vi "RUN.vi"(8 "error in (no error)":errorcluster, 11 "SPARC4_AC in":refnum<class "S4ACS_GUI.lvclass">) -> (0 "error out":errorcluster, 3 "SPARC4_AC out":refnum<class "S4ACS_GUI.lvclass">)   [LabVIEW 2018, in "S4ACS_GUI.lvclass"]
uses:
  S4ACS_GUI.lvclass
  StateMachine/State Machine.lvclass
  Interface/Interface.lvclass
  RxTx/RxTx.lvclass
  SyncBox/Sync Box.lvclass
  Channel Manager/Channel Manager.lvclass
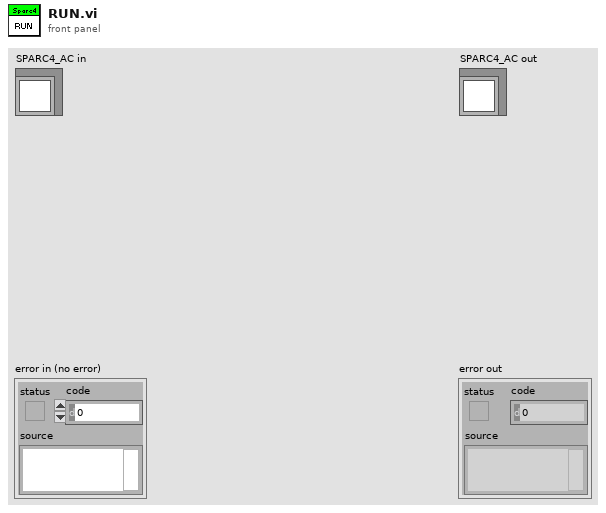
[diagram p1: front panel]
types:
  T1 = cluster{"Image Name":string, "Image Path":string, "# Images":u32, "Exposure Time":dbl, "Pre-amp gain":u8, "Readout Rate":u8, "Vertical Shift Speed":u8, "Acquisition Mode":u8, "Trigger":u8, "Read Mode":u8, "EM Mode":u8, "EM Gain":u16, "Shutter Mode":u8, "Shutter TTL":u8, "Time to open shutter":u16, "Time to close shutter":u16, "Vertical Binning":u16, "Horizontal Binning":u16, "Initial Line":u16, "Initial Column":u16, "Final Line":u16, "Final Column":u16, "Image Name (TEMP)":string, "#img in sequence":u32, "Kinetic Series Length":u32, "Number of Accumulations":u32, "Kinetic Cycle Time":u32, "Frame Transfer":bool, "Vertical Clock Amplitude":u8}
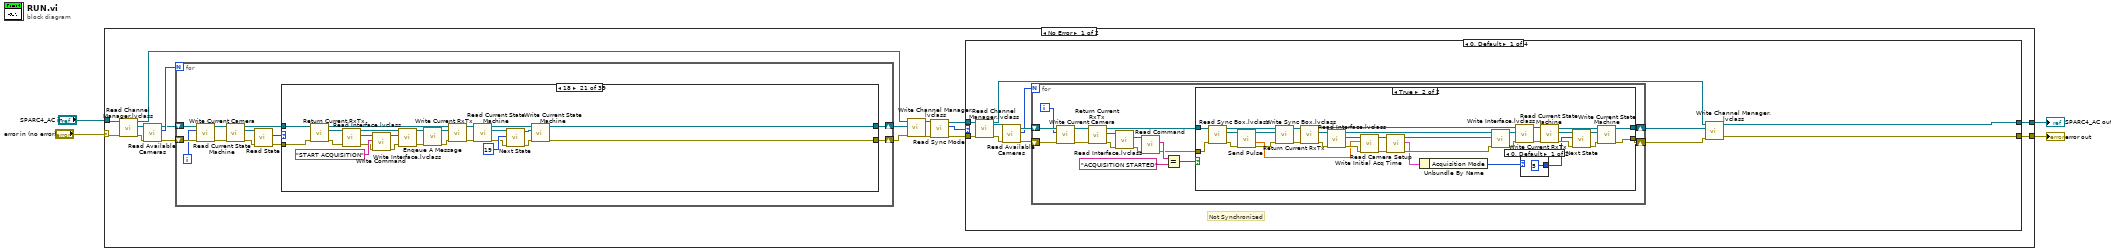
[diagram p0: block diagram]
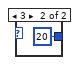
[diagram p3: hidden frame]
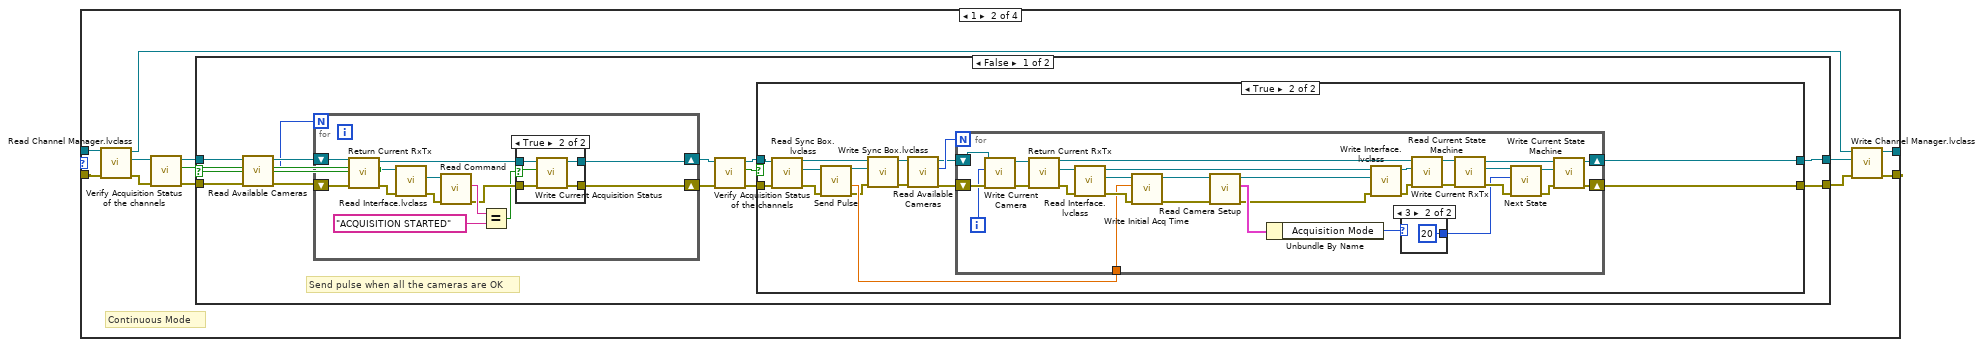
[diagram p4: hidden frame]
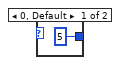
[diagram p6: hidden frame]
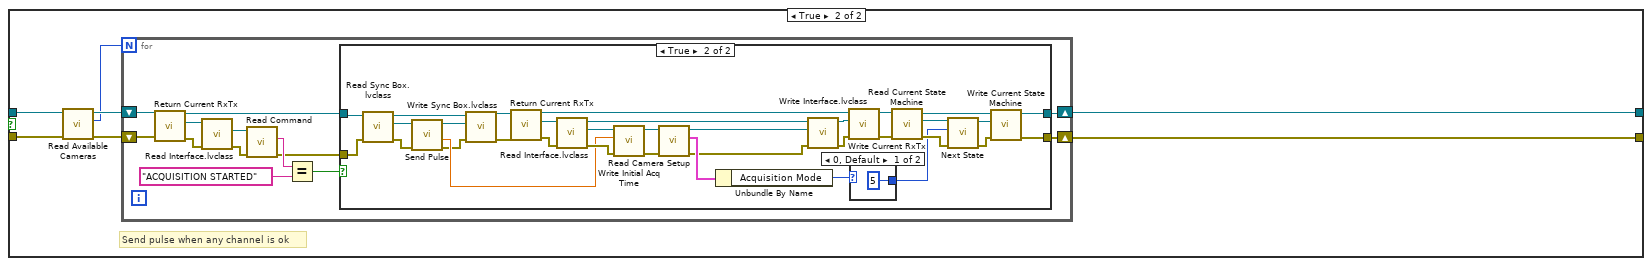
[diagram p8: hidden frame]
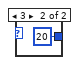
[diagram p10: hidden frame]
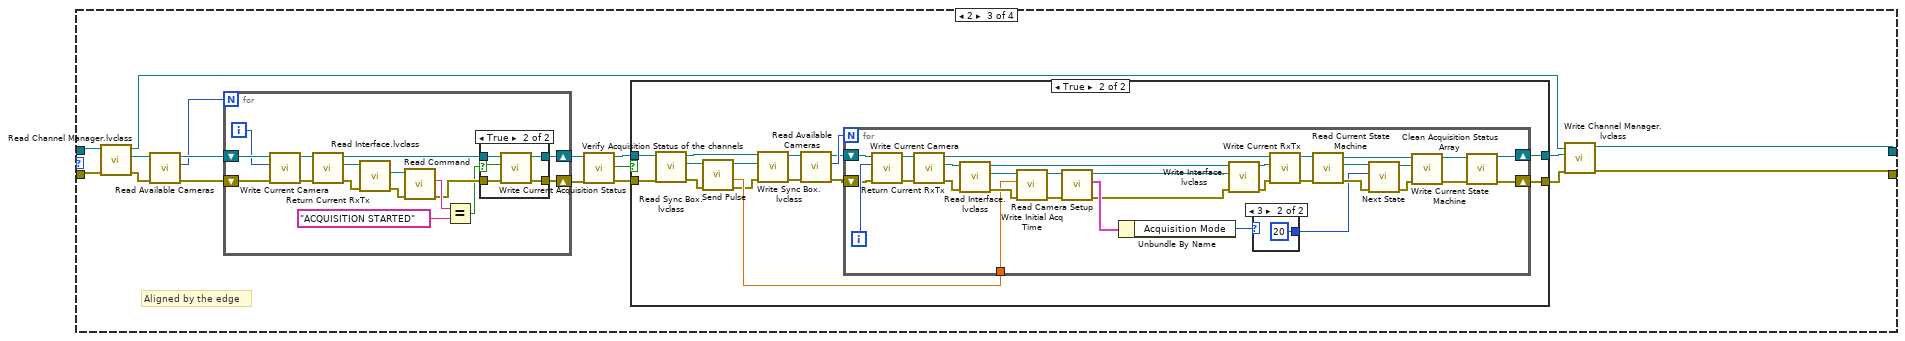
[diagram p11: hidden frame]
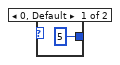
[diagram p13: hidden frame]
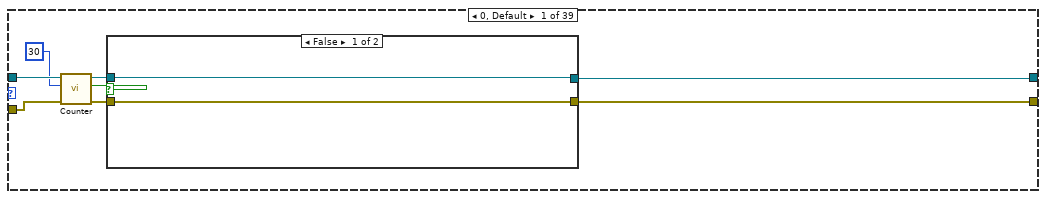
[diagram p16: hidden frame]
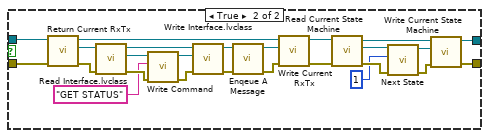
[diagram p17: hidden frame]
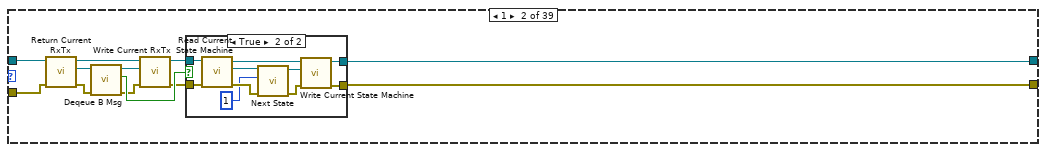
[diagram p18: hidden frame]
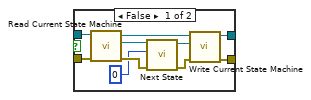
[diagram p19: hidden frame]
diagram:
  n1 = case shown="No Error" "error in (no error)" {
    selector: "error in (no error)" -> [w21 w1413]
    tunnel: [w16 w1414] -> w2
    tunnel: "SPARC4_AC in" -> [w20 w1414]
    tunnel: [w15 w1413] -> w1
    frame No Error {
      n2 = call-dynamic "Read Channel Manager.lvclass.vi"("error in (no error)"=w21, "SPARC4_AC in"=w20) -> ("error out"=w8:errorcluster, "Channel Manager.lvclass"=w9:refnum<class "Channel Manager.lvclass">, "SPARC4_AC out"=w12:refnum<class "S4ACS_GUI.lvclass">)  [unwired: 7 in]
      n3 = call-dynamic "Read Available Cameras.vi"("error in (no error)"=w8, "Channel Manager in"=w9) -> ("error out"=w5:errorcluster, "Available Cameras"=w7:u8, "Channel Manager out"=w6:refnum<class "Channel Manager.lvclass">)  [unwired: 7 in]
      n4 = for {
        N: w7 -> [_]
        shift-right: [w337] -> w13
        shift-left: w6 -> [w334]
        shift-right: [w338] -> w14
        shift-left: w5 -> [w333]
        i -> [w332]
        n5 = call-dynamic "Write Current Camera.vi"("error in (no error)"=w333, "Current Camera"=w332, "Channel Manager in"=w334) -> ("error out"=w336:errorcluster, "Channel Manager out"=w335:refnum<class "Channel Manager.lvclass">)  [unwired: 7 in]
        n6 = call "Read Current State Machine.vi"("error in (no error)"=w336, "Channel Manager in"=w335) -> ("error out"=w340:errorcluster, "State Machine.lvclass"=w341:refnum<class "State Machine.lvclass">, "Channel Manager out"=w339:refnum<class "Channel Manager.lvclass">)  [unwired: 7 in]
        n7 = call-dynamic "Read State.vi"("error in (no error)"=w340, "State Machine in"=w341) -> ("error out"=w342:errorcluster, "State"=w343:u8)  [unwired: 7 in, 1 out]
        n8 = case shown="18" w343 {
          tunnel: w342 -> [w349 w389 w411 w429 w451 w468 w506 w520 w573 w598 w655 w665 w706 w724 w746 w771 w815 w830 w858 w863 w890 w915 w948 w974 w998 w1024 w1049 w1073 w1108 w1145 w1188 w1198 w1227 w1263 w1286 w1305 w1342 w1366 w1391]
          tunnel: w339 -> [w346 w390 w412 w430 w450 w467 w507 w521 w574 w597 w656 w664 w707 w725 w747 w772 w816 w831 w859 w862 w889 w914 w947 w973 w999 w1023 w1050 w1072 w1109 w1146 w1187 w1197 w1228 w1262 w1287 w1306 w1343 w1367 w1392]
          tunnel: [w351 w380 w412 w414 w440 w465 w493 w516 w560 w596 w644 w662 w698 w714 w733 w770 w804 w828 w859 w861 w888 w913 w937 w972 w997 w1022 w1047 w1071 w1107 w1144 w1186 w1196 w1226 w1261 w1285 w1304 w1341 w1365 w1390] -> w337
          tunnel: [w350 w379 w411 w413 w441 w466 w492 w515 w559 w595 w643 w663 w697 w713 w732 w769 w803 w827 w858 w860 w887 w912 w923 w971 w996 w1021 w1048 w1070 w1106 w1143 w1185 w1195 w1225 w1260 w1284 w1303 w1340 w1364 w1389] -> w338
          frame 0, Default {
            n9 = call "Counter.vi"("error in (no error)"=w349, "Interval"=u16 30, "Channel Manager in"=w346) -> ("error out"=w348:errorcluster, "Timeout?"=w345:bool, "Channel Manager out"=w347:refnum<class "Channel Manager.lvclass">)  [unwired: 6 in]
            n10 = case shown="False" w345 {
              tunnel: [w353 w357] -> w351
              tunnel: [w352 w356] -> w350
              tunnel: w348 -> [w352 w355]
              tunnel: w347 -> [w353 w354]
              frame False {
              }
              frame True {
                n11 = call "Return Current RxTx.vi"("error in (no error)"=w355, "Channel Manager in"=w354) -> ("error out"=w369:errorcluster, "RxTx"=w370:refnum<class "RxTx.lvclass">, "Channel Manager out"=w368:refnum<class "Channel Manager.lvclass">)  [unwired: 7 in]
                n12 = call-dynamic "Read Interface.lvclass.vi"("error in (no error)"=w369, "RxTx in"=w370) -> ("error out"=w377:errorcluster, "Interface.lvclass"=w378:refnum<class "Interface.lvclass">, "RxTx out"=w374:refnum<class "RxTx.lvclass">)  [unwired: 7 in]
                n13 = call "Write Command.vi"("error in (no error)"=w377, "Command"="GET STATUS", "Interface in"=w378) -> ("error out"=w376:errorcluster, "Interface out"=w375:refnum<class "Interface.lvclass">)  [unwired: 7 in]
                n14 = call-dynamic "Write Interface.lvclass.vi"("error in (no error)"=w376, "Interface.lvclass"=w375, "RxTx in"=w374) -> ("error out"=w372:errorcluster, "RxTx out"=w371:refnum<class "RxTx.lvclass">)  [unwired: 7 in]
                n15 = call "Enqeue A Message.vi"("error in (no error)"=w372, "RxTx in"=w371) -> ("error out"=w366:errorcluster, "RxTx out"=w367:refnum<class "RxTx.lvclass">)  [unwired: 8 in]
                n16 = call "Write Current RxTx.vi"("error in (no error)"=w366, "RxTx"=w367, "Channel Manager in"=w368) -> ("error out"=w359:errorcluster, "Channel Manager out"=w358:refnum<class "Channel Manager.lvclass">)  [unwired: 7 in]
                n17 = call "Read Current State Machine.vi"("error in (no error)"=w359, "Channel Manager in"=w358) -> ("error out"=w361:errorcluster, "State Machine.lvclass"=w362:refnum<class "State Machine.lvclass">, "Channel Manager out"=w365:refnum<class "Channel Manager.lvclass">)  [unwired: 7 in]
                n18 = call "Next State.vi"("error in (no error)"=w361, "New_State"=u32 1, "State Machine in"=w362) -> ("error out"=w363:errorcluster, "State Machine out"=w364:refnum<class "State Machine.lvclass">)  [unwired: 7 in]
                n19 = call "Write Current State Machine.vi"("error in (no error)"=w363, "State Machine.lvclass"=w364, "Channel Manager in"=w365) -> ("error out"=w356:errorcluster, "Channel Manager out"=w357:refnum<class "Channel Manager.lvclass">)  [unwired: 7 in]
              }
            }
          }
          frame 1 {
            n20 = call "Return Current RxTx.vi"("error in (no error)"=w389, "Channel Manager in"=w390) -> ("error out"=w387:errorcluster, "RxTx"=w388:refnum<class "RxTx.lvclass">, "Channel Manager out"=w383:refnum<class "Channel Manager.lvclass">)  [unwired: 7 in]
            n21 = call "Deqeue B Msg.vi"("error in (no error)"=w387, "RxTx in"=w388) -> ("error out"=w385:errorcluster, "timeout?"=w386:bool, "RxTx out"=w384:refnum<class "RxTx.lvclass">)  [unwired: 7 in]
            n22 = call "Write Current RxTx.vi"("error in (no error)"=w385, "RxTx"=w384, "Channel Manager in"=w383) -> ("error out"=w381:errorcluster, "Channel Manager out"=w382:refnum<class "Channel Manager.lvclass">)  [unwired: 7 in]
            n23 = case shown="True" w386 {
              tunnel: w382 -> [w393 w404]
              tunnel: w381 -> [w394 w403]
              tunnel: [w392 w402] -> w380
              tunnel: [w391 w401] -> w379
              frame False {
                n24 = call "Read Current State Machine.vi"("error in (no error)"=w394, "Channel Manager in"=w393) -> ("error out"=w396:errorcluster, "State Machine.lvclass"=w397:refnum<class "State Machine.lvclass">, "Channel Manager out"=w400:refnum<class "Channel Manager.lvclass">)  [unwired: 7 in]
                n25 = call "Next State.vi"("error in (no error)"=w396, "New_State"=u32 0, "State Machine in"=w397) -> ("error out"=w398:errorcluster, "State Machine out"=w399:refnum<class "State Machine.lvclass">)  [unwired: 7 in]
                n26 = call "Write Current State Machine.vi"("error in (no error)"=w398, "State Machine.lvclass"=w399, "Channel Manager in"=w400) -> ("error out"=w391:errorcluster, "Channel Manager out"=w392:refnum<class "Channel Manager.lvclass">)  [unwired: 7 in]
              }
              frame True {
                n27 = call "Read Current State Machine.vi"("error in (no error)"=w403, "Channel Manager in"=w404) -> ("error out"=w406:errorcluster, "State Machine.lvclass"=w407:refnum<class "State Machine.lvclass">, "Channel Manager out"=w410:refnum<class "Channel Manager.lvclass">)  [unwired: 7 in]
                n28 = call "Next State.vi"("error in (no error)"=w406, "New_State"=u32 1, "State Machine in"=w407) -> ("error out"=w408:errorcluster, "State Machine out"=w409:refnum<class "State Machine.lvclass">)  [unwired: 7 in]
                n29 = call "Write Current State Machine.vi"("error in (no error)"=w408, "State Machine.lvclass"=w409, "Channel Manager in"=w410) -> ("error out"=w401:errorcluster, "Channel Manager out"=w402:refnum<class "Channel Manager.lvclass">)  [unwired: 7 in]
              }
            }
          }
          frame 99 {
          }
          frame 2 {
            # "Limpa array de status de aquisição.\nNecessário para o modo de sincronização contínuo"
            n30 = call "Return Current RxTx.vi"("error in (no error)"=w429, "Channel Manager in"=w430) -> ("error out"=w427:errorcluster, "RxTx"=w428:refnum<class "RxTx.lvclass">, "Channel Manager out"=w424:refnum<class "Channel Manager.lvclass">)  [unwired: 7 in]
            n31 = call-dynamic "Read Interface.lvclass.vi"("error in (no error)"=w427, "RxTx in"=w428) -> ("error out"=w437:errorcluster, "Interface.lvclass"=w438:refnum<class "Interface.lvclass">, "RxTx out"=w432:refnum<class "RxTx.lvclass">)  [unwired: 7 in]
            n32 = call "Write Command.vi"("error in (no error)"=w437, "Command"="WRITE CAMERA SETUP", "Interface in"=w438) -> ("error out"=w434:errorcluster, "Interface out"=w433:refnum<class "Interface.lvclass">)  [unwired: 7 in]
            n33 = call-dynamic "Write Interface.lvclass.vi"("error in (no error)"=w434, "Interface.lvclass"=w433, "RxTx in"=w432) -> ("error out"=w436:errorcluster, "RxTx out"=w435:refnum<class "RxTx.lvclass">)  [unwired: 7 in]
            n34 = call "Enqeue A Message.vi"("error in (no error)"=w436, "RxTx in"=w435) -> ("error out"=w426:errorcluster, "RxTx out"=w425:refnum<class "RxTx.lvclass">)  [unwired: 8 in]
            n35 = call "Write Current RxTx.vi"("error in (no error)"=w426, "RxTx"=w425, "Channel Manager in"=w424) -> ("error out"=w423:errorcluster, "Channel Manager out"=w422:refnum<class "Channel Manager.lvclass">)  [unwired: 7 in]
            n36 = call "Read Current State Machine.vi"("error in (no error)"=w423, "Channel Manager in"=w422) -> ("error out"=w420:errorcluster, "State Machine.lvclass"=w421:refnum<class "State Machine.lvclass">, "Channel Manager out"=w417:refnum<class "Channel Manager.lvclass">)  [unwired: 7 in]
            n37 = call "Next State.vi"("error in (no error)"=w420, "New_State"=u32 3, "State Machine in"=w421) -> ("error out"=w419:errorcluster, "State Machine out"=w418:refnum<class "State Machine.lvclass">)  [unwired: 7 in]
            n38 = call "Write Current State Machine.vi"("error in (no error)"=w419, "State Machine.lvclass"=w418, "Channel Manager in"=w417) -> ("error out"=w416:errorcluster, "Channel Manager out"=w415:refnum<class "Channel Manager.lvclass">)  [unwired: 7 in]
            n39 = call "Clean Acquisition Status Array.vi"("error in (no error)"=w416, "Channel Manager in"=w415) -> ("error out"=w413:errorcluster, "Channel Manager out"=w414:refnum<class "Channel Manager.lvclass">)  [unwired: 8 in]
          }
          frame 3 {
            n40 = call "Return Current RxTx.vi"("error in (no error)"=w451, "Channel Manager in"=w450) -> ("error out"=w455:errorcluster, "RxTx"=w456:refnum<class "RxTx.lvclass">, "Channel Manager out"=w452:refnum<class "Channel Manager.lvclass">)  [unwired: 7 in]
            n41 = call-dynamic "Read Interface.lvclass.vi"("error in (no error)"=w455, "RxTx in"=w456) -> ("error out"=w462:errorcluster, "Interface.lvclass"=w463:refnum<class "Interface.lvclass">, "RxTx out"=w457:refnum<class "RxTx.lvclass">)  [unwired: 7 in]
            n42 = call "Write Command.vi"("error in (no error)"=w462, "Command"="START ACQUISITION", "Interface in"=w463) -> ("error out"=w459:errorcluster, "Interface out"=w458:refnum<class "Interface.lvclass">)  [unwired: 7 in]
            n43 = call-dynamic "Write Interface.lvclass.vi"("error in (no error)"=w459, "Interface.lvclass"=w458, "RxTx in"=w457) -> ("error out"=w461:errorcluster, "RxTx out"=w460:refnum<class "RxTx.lvclass">)  [unwired: 7 in]
            n44 = call "Enqeue A Message.vi"("error in (no error)"=w461, "RxTx in"=w460) -> ("error out"=w454:errorcluster, "RxTx out"=w453:refnum<class "RxTx.lvclass">)  [unwired: 8 in]
            n45 = call "Write Current RxTx.vi"("error in (no error)"=w454, "RxTx"=w453, "Channel Manager in"=w452) -> ("error out"=w444:errorcluster, "Channel Manager out"=w443:refnum<class "Channel Manager.lvclass">)  [unwired: 7 in]
            n46 = call "Read Current State Machine.vi"("error in (no error)"=w444, "Channel Manager in"=w443) -> ("error out"=w448:errorcluster, "State Machine.lvclass"=w447:refnum<class "State Machine.lvclass">, "Channel Manager out"=w442:refnum<class "Channel Manager.lvclass">)  [unwired: 7 in]
            n47 = call "Next State.vi"("error in (no error)"=w448, "New_State"=u32 4, "State Machine in"=w447) -> ("error out"=w446:errorcluster, "State Machine out"=w445:refnum<class "State Machine.lvclass">)  [unwired: 7 in]
            n48 = call "Write Current State Machine.vi"("error in (no error)"=w446, "State Machine.lvclass"=w445, "Channel Manager in"=w442) -> ("error out"=w441:errorcluster, "Channel Manager out"=w440:refnum<class "Channel Manager.lvclass">)  [unwired: 7 in]
          }
          frame 4 {
            n49 = call "Return Current RxTx.vi"("error in (no error)"=w468, "Channel Manager in"=w467) -> ("error out"=w472:errorcluster, "RxTx"=w473:refnum<class "RxTx.lvclass">, "Channel Manager out"=w474:refnum<class "Channel Manager.lvclass">)  [unwired: 7 in]
            n50 = call "Deqeue B Msg.vi"("error in (no error)"=w472, "RxTx in"=w473) -> ("error out"=w475:errorcluster, "timeout?"=w469:bool, "RxTx out"=w476:refnum<class "RxTx.lvclass">)  [unwired: 7 in]
            n51 = call "Write Current RxTx.vi"("error in (no error)"=w475, "RxTx"=w476, "Channel Manager in"=w474) -> ("error out"=w471:errorcluster, "Channel Manager out"=w470:refnum<class "Channel Manager.lvclass">)  [unwired: 7 in]
            n52 = case shown="True" w469 {
              tunnel: w471 -> [w477 w482]
              tunnel: w470 -> [w478 w481]
              tunnel: [w478 w480] -> w465
              tunnel: [w477 w479] -> w466
              frame False {
              }
              frame True {
                n53 = call "Read Current State Machine.vi"("error in (no error)"=w482, "Channel Manager in"=w481) -> ("error out"=w484:errorcluster, "State Machine.lvclass"=w485:refnum<class "State Machine.lvclass">, "Channel Manager out"=w488:refnum<class "Channel Manager.lvclass">)  [unwired: 7 in]
                n54 = call "Next State.vi"("error in (no error)"=w484, "New_State"=u32 4, "State Machine in"=w485) -> ("error out"=w486:errorcluster, "State Machine out"=w487:refnum<class "State Machine.lvclass">)  [unwired: 7 in]
                n55 = call "Write Current State Machine.vi"("error in (no error)"=w486, "State Machine.lvclass"=w487, "Channel Manager in"=w488) -> ("error out"=w479:errorcluster, "Channel Manager out"=w480:refnum<class "Channel Manager.lvclass">)  [unwired: 7 in]
              }
            }
          }
          frame 5 {
            n56 = call "Return Current RxTx.vi"("error in (no error)"=w506, "Channel Manager in"=w507) -> ("error out"=w504:errorcluster, "RxTx"=w505:refnum<class "RxTx.lvclass">, "Channel Manager out"=w501:refnum<class "Channel Manager.lvclass">)  [unwired: 7 in]
            n57 = call-dynamic "Read Interface.lvclass.vi"("error in (no error)"=w504, "RxTx in"=w505) -> ("error out"=w512:errorcluster, "Interface.lvclass"=w513:refnum<class "Interface.lvclass">, "RxTx out"=w509:refnum<class "RxTx.lvclass">)  [unwired: 7 in]
            n58 = call "Write Command.vi"("error in (no error)"=w512, "Command"="VERIFY ACQUISITION", "Interface in"=w513) -> ("error out"=w490:errorcluster, "Interface out"=w491:refnum<class "Interface.lvclass">)  [unwired: 7 in]
            n59 = call-dynamic "Write Interface.lvclass.vi"("error in (no error)"=w490, "Interface.lvclass"=w491, "RxTx in"=w509) -> ("error out"=w511:errorcluster, "RxTx out"=w510:refnum<class "RxTx.lvclass">)  [unwired: 7 in]
            n60 = call "Enqeue A Message.vi"("error in (no error)"=w511, "RxTx in"=w510) -> ("error out"=w503:errorcluster, "RxTx out"=w502:refnum<class "RxTx.lvclass">)  [unwired: 8 in]
            n61 = call "Write Current RxTx.vi"("error in (no error)"=w503, "RxTx"=w502, "Channel Manager in"=w501) -> ("error out"=w500:errorcluster, "Channel Manager out"=w499:refnum<class "Channel Manager.lvclass">)  [unwired: 7 in]
            n62 = call "Read Current State Machine.vi"("error in (no error)"=w500, "Channel Manager in"=w499) -> ("error out"=w498:errorcluster, "State Machine.lvclass"=w497:refnum<class "State Machine.lvclass">, "Channel Manager out"=w494:refnum<class "Channel Manager.lvclass">)  [unwired: 7 in]
            n63 = call "Next State.vi"("error in (no error)"=w498, "New_State"=u32 6, "State Machine in"=w497) -> ("error out"=w496:errorcluster, "State Machine out"=w495:refnum<class "State Machine.lvclass">)  [unwired: 7 in]
            n64 = call "Write Current State Machine.vi"("error in (no error)"=w496, "State Machine.lvclass"=w495, "Channel Manager in"=w494) -> ("error out"=w492:errorcluster, "Channel Manager out"=w493:refnum<class "Channel Manager.lvclass">)  [unwired: 7 in]
          }
          frame 6 {
            n65 = call "Return Current RxTx.vi"("error in (no error)"=w520, "Channel Manager in"=w521) -> ("error out"=w518:errorcluster, "RxTx"=w519:refnum<class "RxTx.lvclass">, "Channel Manager out"=w517:refnum<class "Channel Manager.lvclass">)  [unwired: 7 in]
            n66 = call "Deqeue B Msg.vi"("error in (no error)"=w518, "RxTx in"=w519) -> ("error out"=w523:errorcluster, "timeout?"=w514:bool, "RxTx out"=w522:refnum<class "RxTx.lvclass">)  [unwired: 7 in]
            n67 = case shown="False" w514 {
              tunnel: w523 -> [w541 w553]
              tunnel: w522 -> [w540 w552]
              tunnel: w517 -> [w535 w551]
              tunnel: [w527 w548] -> w516
              tunnel: [w526 w547] -> w515
              frame False {
                n68 = call-dynamic "Read Interface.lvclass.vi"("error in (no error)"=w541, "RxTx in"=w540) -> ("error out"=w538:errorcluster, "Interface.lvclass"=w539:refnum<class "Interface.lvclass">, "RxTx out"=w537:refnum<class "RxTx.lvclass">)  [unwired: 7 in]
                n69 = call "Read Command.vi"("error in (no error)"=w538, "Interface in"=w539) -> ("error out"=w536:errorcluster, "Command"=w525:string)  [unwired: 7 in, 1 out]
                n70 = call "Write Current RxTx.vi"("error in (no error)"=w536, "RxTx"=w537, "Channel Manager in"=w535) -> ("error out"=w534:errorcluster, "Channel Manager out"=w533:refnum<class "Channel Manager.lvclass">)  [unwired: 7 in]
                n71 = case shown="\"ACQUISITION COMPLETED\"" w525 {
                  tunnel: [u32 4 ("New_State") u32 7 ("New_State") u32 9 ("New_State")] -> w524
                  frame "False", Default {
                  }
                  frame "ACQUIRING" {
                  }
                  frame "ACQUISITION COMPLETED" {
                  }
                }
                n72 = call "Read Current State Machine.vi"("error in (no error)"=w534, "Channel Manager in"=w533) -> ("error out"=w531:errorcluster, "State Machine.lvclass"=w532:refnum<class "State Machine.lvclass">, "Channel Manager out"=w528:refnum<class "Channel Manager.lvclass">)  [unwired: 7 in]
                n73 = call "Next State.vi"("error in (no error)"=w531, "New_State"=w524, "State Machine in"=w532) -> ("error out"=w530:errorcluster, "State Machine out"=w529:refnum<class "State Machine.lvclass">)  [unwired: 7 in]
                n74 = call "Write Current State Machine.vi"("error in (no error)"=w530, "State Machine.lvclass"=w529, "Channel Manager in"=w528) -> ("error out"=w526:errorcluster, "Channel Manager out"=w527:refnum<class "Channel Manager.lvclass">)  [unwired: 7 in]
              }
              frame True {
                n75 = call "Write Current RxTx.vi"("error in (no error)"=w553, "RxTx"=w552, "Channel Manager in"=w551) -> ("error out"=w550:errorcluster, "Channel Manager out"=w549:refnum<class "Channel Manager.lvclass">)  [unwired: 7 in]
                n76 = call "Read Current State Machine.vi"("error in (no error)"=w550, "Channel Manager in"=w549) -> ("error out"=w546:errorcluster, "State Machine.lvclass"=w556:refnum<class "State Machine.lvclass">, "Channel Manager out"=w554:refnum<class "Channel Manager.lvclass">)  [unwired: 7 in]
                n77 = call "Next State.vi"("error in (no error)"=w546, "New_State"=u32 6, "State Machine in"=w556) -> ("error out"=w557:errorcluster, "State Machine out"=w555:refnum<class "State Machine.lvclass">)  [unwired: 7 in]
                n78 = call "Write Current State Machine.vi"("error in (no error)"=w557, "State Machine.lvclass"=w555, "Channel Manager in"=w554) -> ("error out"=w547:errorcluster, "Channel Manager out"=w548:refnum<class "Channel Manager.lvclass">)  [unwired: 7 in]
              }
            }
          }
          frame 7 {
            n79 = call "Return Current RxTx.vi"("error in (no error)"=w573, "Channel Manager in"=w574) -> ("error out"=w571:errorcluster, "RxTx"=w572:refnum<class "RxTx.lvclass">, "Channel Manager out"=w562:refnum<class "Channel Manager.lvclass">)  [unwired: 7 in]
            n80 = call-dynamic "Read Interface.lvclass.vi"("error in (no error)"=w571, "RxTx in"=w572) -> ("error out"=w579:errorcluster, "Interface.lvclass"=w580:refnum<class "Interface.lvclass">, "RxTx out"=w575:refnum<class "RxTx.lvclass">)  [unwired: 7 in]
            n81 = call-dynamic "Read Abort.vi"("error in (no error)"=w579, "Interface in"=w580) -> ("error out"=w576:errorcluster, "Abort"=w578:bool, "Interface out"=w577:refnum<class "Interface.lvclass">)  [unwired: 7 in]
            n82 = case shown="False" w578 {
              tunnel: w577 -> [_ w593]
              tunnel: w576 -> [w582 w592]
              tunnel: w575 -> [w583 w589]
              tunnel: [w583 w586] -> w563
              tunnel: [w582 w585] -> w561
              tunnel: [5 8] -> w558
              frame False {
              }
              frame True {
                n83 = call "Write Command.vi"("error in (no error)"=w592, "Command"="ABORT ACQUISITION", "Interface in"=w593) -> ("error out"=w588:errorcluster, "Interface out"=w587:refnum<class "Interface.lvclass">)  [unwired: 7 in]
                n84 = call-dynamic "Write Interface.lvclass.vi"("error in (no error)"=w588, "Interface.lvclass"=w587, "RxTx in"=w589) -> ("error out"=w590:errorcluster, "RxTx out"=w591:refnum<class "RxTx.lvclass">)  [unwired: 7 in]
                n85 = call "Enqeue A Message.vi"("error in (no error)"=w590, "RxTx in"=w591) -> ("error out"=w585:errorcluster, "RxTx out"=w586:refnum<class "RxTx.lvclass">)  [unwired: 8 in]
              }
            }
            n86 = call "Write Current RxTx.vi"("error in (no error)"=w561, "RxTx"=w563, "Channel Manager in"=w562) -> ("error out"=w570:errorcluster, "Channel Manager out"=w569:refnum<class "Channel Manager.lvclass">)  [unwired: 7 in]
            n87 = call "Read Current State Machine.vi"("error in (no error)"=w570, "Channel Manager in"=w569) -> ("error out"=w567:errorcluster, "State Machine.lvclass"=w568:refnum<class "State Machine.lvclass">, "Channel Manager out"=w564:refnum<class "Channel Manager.lvclass">)  [unwired: 7 in]
            n88 = call "Next State.vi"("error in (no error)"=w567, "New_State"=w558, "State Machine in"=w568) -> ("error out"=w566:errorcluster, "State Machine out"=w565:refnum<class "State Machine.lvclass">)  [unwired: 7 in]
            n89 = call "Write Current State Machine.vi"("error in (no error)"=w566, "State Machine.lvclass"=w565, "Channel Manager in"=w564) -> ("error out"=w559:errorcluster, "Channel Manager out"=w560:refnum<class "Channel Manager.lvclass">)  [unwired: 7 in]
          }
          frame 8 {
            n90 = call "Return Current RxTx.vi"("error in (no error)"=w598, "Channel Manager in"=w597) -> ("error out"=w605:errorcluster, "RxTx"=w606:refnum<class "RxTx.lvclass">, "Channel Manager out"=w601:refnum<class "Channel Manager.lvclass">)  [unwired: 7 in]
            n91 = call "Deqeue B Msg.vi"("error in (no error)"=w605, "RxTx in"=w606) -> ("error out"=w603:errorcluster, "timeout?"=w604:bool, "RxTx out"=w602:refnum<class "RxTx.lvclass">)  [unwired: 7 in]
            n92 = call "Write Current RxTx.vi"("error in (no error)"=w603, "RxTx"=w602, "Channel Manager in"=w601) -> ("error out"=w599:errorcluster, "Channel Manager out"=w600:refnum<class "Channel Manager.lvclass">)  [unwired: 7 in]
            n93 = case shown="False" w604 {
              tunnel: w600 -> [w609 w620]
              tunnel: w599 -> [w610 w619]
              tunnel: [w608 w618] -> w596
              tunnel: [w607 w617] -> w595
              frame False {
                n94 = call "Read Current State Machine.vi"("error in (no error)"=w610, "Channel Manager in"=w609) -> ("error out"=w612:errorcluster, "State Machine.lvclass"=w613:refnum<class "State Machine.lvclass">, "Channel Manager out"=w616:refnum<class "Channel Manager.lvclass">)  [unwired: 7 in]
                n95 = call "Next State.vi"("error in (no error)"=w612, "New_State"=u32 0, "State Machine in"=w613) -> ("error out"=w614:errorcluster, "State Machine out"=w615:refnum<class "State Machine.lvclass">)  [unwired: 7 in]
                n96 = call "Write Current State Machine.vi"("error in (no error)"=w614, "State Machine.lvclass"=w615, "Channel Manager in"=w616) -> ("error out"=w607:errorcluster, "Channel Manager out"=w608:refnum<class "Channel Manager.lvclass">)  [unwired: 7 in]
              }
              frame True {
                n97 = call "Read Current State Machine.vi"("error in (no error)"=w619, "Channel Manager in"=w620) -> ("error out"=w622:errorcluster, "State Machine.lvclass"=w623:refnum<class "State Machine.lvclass">, "Channel Manager out"=w626:refnum<class "Channel Manager.lvclass">)  [unwired: 7 in]
                n98 = call "Next State.vi"("error in (no error)"=w622, "New_State"=u32 8, "State Machine in"=w623) -> ("error out"=w624:errorcluster, "State Machine out"=w625:refnum<class "State Machine.lvclass">)  [unwired: 7 in]
                n99 = call "Write Current State Machine.vi"("error in (no error)"=w624, "State Machine.lvclass"=w625, "Channel Manager in"=w626) -> ("error out"=w617:errorcluster, "Channel Manager out"=w618:refnum<class "Channel Manager.lvclass">)  [unwired: 7 in]
              }
            }
          }
          frame 9 {
            n100 = call "Return Current RxTx.vi"("error in (no error)"=w655, "Channel Manager in"=w656) -> ("error out"=w653:errorcluster, "RxTx"=w654:refnum<class "RxTx.lvclass">, "Channel Manager out"=w652:refnum<class "Channel Manager.lvclass">)  [unwired: 7 in]
            n101 = call-dynamic "Read Interface.lvclass.vi"("error in (no error)"=w653, "RxTx in"=w654) -> ("error out"=w639:errorcluster, "Interface.lvclass"=w640:refnum<class "Interface.lvclass">, "RxTx out"=w657:refnum<class "RxTx.lvclass">)  [unwired: 7 in]
            n102 = call "Write Command.vi"("error in (no error)"=w639, "Command"="CREATE CONCRETE PRODUCT SINGLE", "Interface in"=w640) -> ("error out"=w659:errorcluster, "Interface out"=w658:refnum<class "Interface.lvclass">)  [unwired: 7 in]
            n103 = call-dynamic "Write Interface.lvclass.vi"("error in (no error)"=w659, "Interface.lvclass"=w658, "RxTx in"=w657) -> ("error out"=w661:errorcluster, "RxTx out"=w660:refnum<class "RxTx.lvclass">)  [unwired: 7 in]
            n104 = call "Enqeue A Message.vi"("error in (no error)"=w661, "RxTx in"=w660) -> ("error out"=w635:errorcluster, "RxTx out"=w634:refnum<class "RxTx.lvclass">)  [unwired: 8 in]
            n105 = call-dynamic "Read Interface.lvclass.vi"("error in (no error)"=w635, "RxTx in"=w634) -> ("error out"=w633:errorcluster, "Interface.lvclass"=w632:refnum<class "Interface.lvclass">, "RxTx out"=w631:refnum<class "RxTx.lvclass">)  [unwired: 7 in]
            n106 = call "Write Command.vi"("error in (no error)"=w633, "Command"="SAVE IMAGE SINGLE", "Interface in"=w632) -> ("error out"=w637:errorcluster, "Interface out"=w638:refnum<class "Interface.lvclass">)  [unwired: 7 in]
            n107 = call-dynamic "Write Interface.lvclass.vi"("error in (no error)"=w637, "Interface.lvclass"=w638, "RxTx in"=w631) -> ("error out"=w636:errorcluster, "RxTx out"=w630:refnum<class "RxTx.lvclass">)  [unwired: 7 in]
            n108 = call "Enqeue A Message.vi"("error in (no error)"=w636, "RxTx in"=w630) -> ("error out"=w628:errorcluster, "RxTx out"=w629:refnum<class "RxTx.lvclass">)  [unwired: 8 in]
            n109 = call "Write Current RxTx.vi"("error in (no error)"=w628, "RxTx"=w629, "Channel Manager in"=w652) -> ("error out"=w646:errorcluster, "Channel Manager out"=w645:refnum<class "Channel Manager.lvclass">)  [unwired: 7 in]
            n110 = call "Read Current State Machine.vi"("error in (no error)"=w646, "Channel Manager in"=w645) -> ("error out"=w650:errorcluster, "State Machine.lvclass"=w651:refnum<class "State Machine.lvclass">, "Channel Manager out"=w647:refnum<class "Channel Manager.lvclass">)  [unwired: 7 in]
            n111 = call "Next State.vi"("error in (no error)"=w650, "New_State"=10, "State Machine in"=w651) -> ("error out"=w649:errorcluster, "State Machine out"=w648:refnum<class "State Machine.lvclass">)  [unwired: 7 in]
            n112 = call "Write Current State Machine.vi"("error in (no error)"=w649, "State Machine.lvclass"=w648, "Channel Manager in"=w647) -> ("error out"=w643:errorcluster, "Channel Manager out"=w644:refnum<class "Channel Manager.lvclass">)  [unwired: 7 in]
          }
          frame 10 {
            n113 = call "Return Current RxTx.vi"("error in (no error)"=w665, "Channel Manager in"=w664) -> ("error out"=w670:errorcluster, "RxTx"=w671:refnum<class "RxTx.lvclass">, "Channel Manager out"=w672:refnum<class "Channel Manager.lvclass">)  [unwired: 7 in]
            n114 = call "Deqeue B Msg.vi"("error in (no error)"=w670, "RxTx in"=w671) -> ("error out"=w669:errorcluster, "timeout?"=w673:bool, "RxTx out"=w668:refnum<class "RxTx.lvclass">)  [unwired: 7 in]
            n115 = call "Write Current RxTx.vi"("error in (no error)"=w669, "RxTx"=w668, "Channel Manager in"=w672) -> ("error out"=w667:errorcluster, "Channel Manager out"=w666:refnum<class "Channel Manager.lvclass">)  [unwired: 7 in]
            n116 = case shown="False" w673 {
              tunnel: w666 -> [w676 w688]
              tunnel: w667 -> [w677 w687]
              tunnel: [w675 w685] -> w662
              tunnel: [w674 w684] -> w663
              frame False {
                n117 = call "Read Current State Machine.vi"("error in (no error)"=w677, "Channel Manager in"=w676) -> ("error out"=w680:errorcluster, "State Machine.lvclass"=w679:refnum<class "State Machine.lvclass">, "Channel Manager out"=w683:refnum<class "Channel Manager.lvclass">)  [unwired: 7 in]
                n118 = call "Next State.vi"("error in (no error)"=w680, "New_State"=u32 11, "State Machine in"=w679) -> ("error out"=w681:errorcluster, "State Machine out"=w682:refnum<class "State Machine.lvclass">)  [unwired: 7 in]
                n119 = call "Write Current State Machine.vi"("error in (no error)"=w681, "State Machine.lvclass"=w682, "Channel Manager in"=w683) -> ("error out"=w674:errorcluster, "Channel Manager out"=w675:refnum<class "Channel Manager.lvclass">)  [unwired: 7 in]
              }
              frame True {
                n120 = call "Read Current State Machine.vi"("error in (no error)"=w687, "Channel Manager in"=w688) -> ("error out"=w690:errorcluster, "State Machine.lvclass"=w689:refnum<class "State Machine.lvclass">, "Channel Manager out"=w693:refnum<class "Channel Manager.lvclass">)  [unwired: 7 in]
                n121 = call "Next State.vi"("error in (no error)"=w690, "New_State"=u32 10, "State Machine in"=w689) -> ("error out"=w691:errorcluster, "State Machine out"=w692:refnum<class "State Machine.lvclass">)  [unwired: 7 in]
                n122 = call "Write Current State Machine.vi"("error in (no error)"=w691, "State Machine.lvclass"=w692, "Channel Manager in"=w693) -> ("error out"=w684:errorcluster, "Channel Manager out"=w685:refnum<class "Channel Manager.lvclass">)  [unwired: 7 in]
              }
            }
          }
          frame 11 {
            n123 = call "Return Current RxTx.vi"("error in (no error)"=w706, "Channel Manager in"=w707) -> ("error out"=w704:errorcluster, "RxTx"=w705:refnum<class "RxTx.lvclass">, "Channel Manager out"=w696:refnum<class "Channel Manager.lvclass">)  [unwired: 7 in]
            n124 = call-dynamic "Read Interface.lvclass.vi"("error in (no error)"=w704, "RxTx in"=w705) -> ("error out"=w709:errorcluster, "Interface.lvclass"=w708:refnum<class "Interface.lvclass">)  [unwired: 7 in, 1 out]
            n125 = call-dynamic "Read # Images.vi"("error in (no error)"=w709, "Interface in"=w708) -> ("error out"=w695:errorcluster, "# Images"=w694:u32)  [unwired: 7 in, 1 out]
            n126 = case shown="0" w694 {
              tunnel: [u32 0 ("New_State") 12] -> w710
              frame 0 {
              }
              frame 1, Default {
              }
            }
            n127 = call "Read Current State Machine.vi"("error in (no error)"=w695, "Channel Manager in"=w696) -> ("error out"=w702:errorcluster, "State Machine.lvclass"=w703:refnum<class "State Machine.lvclass">, "Channel Manager out"=w699:refnum<class "Channel Manager.lvclass">)  [unwired: 7 in]
            n128 = call "Next State.vi"("error in (no error)"=w702, "New_State"=w710, "State Machine in"=w703) -> ("error out"=w701:errorcluster, "State Machine out"=w700:refnum<class "State Machine.lvclass">)  [unwired: 7 in]
            n129 = call "Write Current State Machine.vi"("error in (no error)"=w701, "State Machine.lvclass"=w700, "Channel Manager in"=w699) -> ("error out"=w697:errorcluster, "Channel Manager out"=w698:refnum<class "Channel Manager.lvclass">)  [unwired: 7 in]
          }
          frame 12 {
            n130 = call "Return Current RxTx.vi"("error in (no error)"=w724, "Channel Manager in"=w725) -> ("error out"=w722:errorcluster, "RxTx"=w723:refnum<class "RxTx.lvclass">, "Channel Manager out"=w719:refnum<class "Channel Manager.lvclass">)  [unwired: 7 in]
            n131 = call-dynamic "Read Interface.lvclass.vi"("error in (no error)"=w722, "RxTx in"=w723) -> ("error out"=w726:errorcluster, "Interface.lvclass"=w728:refnum<class "Interface.lvclass">)  [unwired: 7 in, 1 out]
            n132 = call-dynamic "Read Pause Acq.vi"("error in (no error)"=w726, "Interface in"=w728) -> ("error out"=w718:errorcluster, "Pause Acq"=w727:bool)  [unwired: 7 in, 1 out]
            n133 = case shown="False" w727 {
              tunnel: [u32 13 ("# Images") u32 12 ("# Images")] -> w729
              frame False {
              }
              frame True {
              }
            }
            n134 = call "Read Current State Machine.vi"("error in (no error)"=w718, "Channel Manager in"=w719) -> ("error out"=w721:errorcluster, "State Machine.lvclass"=w720:refnum<class "State Machine.lvclass">, "Channel Manager out"=w715:refnum<class "Channel Manager.lvclass">)  [unwired: 7 in]
            n135 = call "Next State.vi"("error in (no error)"=w721, "New_State"=w729, "State Machine in"=w720) -> ("error out"=w717:errorcluster, "State Machine out"=w716:refnum<class "State Machine.lvclass">)  [unwired: 7 in]
            n136 = call "Write Current State Machine.vi"("error in (no error)"=w717, "State Machine.lvclass"=w716, "Channel Manager in"=w715) -> ("error out"=w713:errorcluster, "Channel Manager out"=w714:refnum<class "Channel Manager.lvclass">)  [unwired: 7 in]
          }
          frame 13 {
            n137 = call "Return Current RxTx.vi"("error in (no error)"=w746, "Channel Manager in"=w747) -> ("error out"=w744:errorcluster, "RxTx"=w745:refnum<class "RxTx.lvclass">, "Channel Manager out"=w741:refnum<class "Channel Manager.lvclass">)  [unwired: 7 in]
            n138 = call-dynamic "Read Interface.lvclass.vi"("error in (no error)"=w744, "RxTx in"=w745) -> ("error out"=w752:errorcluster, "Interface.lvclass"=w753:refnum<class "Interface.lvclass">, "RxTx out"=w748:refnum<class "RxTx.lvclass">)  [unwired: 7 in]
            n139 = call-dynamic "Read Stop Acq.vi"("error in (no error)"=w752, "Interface in"=w753) -> ("error out"=w749:errorcluster, "Stop Acq"=w751:bool, "Interface out"=w750:refnum<class "Interface.lvclass">)  [unwired: 7 in]
            n140 = case shown="True" w751 {
              tunnel: w750 -> [_ w764]
              tunnel: w749 -> [w756 w763]
              tunnel: [w755 w759] -> w743
              tunnel: [u32 15 ("# Images") u32 14 ("# Images")] -> w754
              tunnel: w748 -> [w755 w762]
              tunnel: [w756 w758] -> w742
              frame False {
              }
              frame True {
                n141 = call "Write Command.vi"("error in (no error)"=w763, "Command"="STOP ACQUISITION", "Interface in"=w764) -> ("error out"=w761:errorcluster, "Interface out"=w760:refnum<class "Interface.lvclass">)  [unwired: 7 in]
                n142 = call-dynamic "Write Interface.lvclass.vi"("error in (no error)"=w761, "Interface.lvclass"=w760, "RxTx in"=w762) -> ("error out"=w767:errorcluster, "RxTx out"=w766:refnum<class "RxTx.lvclass">)  [unwired: 7 in]
                n143 = call "Enqeue A Message.vi"("error in (no error)"=w767, "RxTx in"=w766) -> ("error out"=w758:errorcluster, "RxTx out"=w759:refnum<class "RxTx.lvclass">)  [unwired: 8 in]
              }
            }
            n144 = call "Write Current RxTx.vi"("error in (no error)"=w742, "RxTx"=w743, "Channel Manager in"=w741) -> ("error out"=w740:errorcluster, "Channel Manager out"=w739:refnum<class "Channel Manager.lvclass">)  [unwired: 7 in]
            n145 = call "Read Current State Machine.vi"("error in (no error)"=w740, "Channel Manager in"=w739) -> ("error out"=w737:errorcluster, "State Machine.lvclass"=w738:refnum<class "State Machine.lvclass">, "Channel Manager out"=w734:refnum<class "Channel Manager.lvclass">)  [unwired: 7 in]
            n146 = call "Next State.vi"("error in (no error)"=w737, "New_State"=w754, "State Machine in"=w738) -> ("error out"=w736:errorcluster, "State Machine out"=w735:refnum<class "State Machine.lvclass">)  [unwired: 7 in]
            n147 = call "Write Current State Machine.vi"("error in (no error)"=w736, "State Machine.lvclass"=w735, "Channel Manager in"=w734) -> ("error out"=w732:errorcluster, "Channel Manager out"=w733:refnum<class "Channel Manager.lvclass">)  [unwired: 7 in]
          }
          frame 14 {
            n148 = call "Return Current RxTx.vi"("error in (no error)"=w771, "Channel Manager in"=w772) -> ("error out"=w777:errorcluster, "RxTx"=w778:refnum<class "RxTx.lvclass">, "Channel Manager out"=w779:refnum<class "Channel Manager.lvclass">)  [unwired: 7 in]
            n149 = call "Deqeue B Msg.vi"("error in (no error)"=w777, "RxTx in"=w778) -> ("error out"=w776:errorcluster, "timeout?"=w780:bool, "RxTx out"=w775:refnum<class "RxTx.lvclass">)  [unwired: 7 in]
            n150 = call "Write Current RxTx.vi"("error in (no error)"=w776, "RxTx"=w775, "Channel Manager in"=w779) -> ("error out"=w774:errorcluster, "Channel Manager out"=w773:refnum<class "Channel Manager.lvclass">)  [unwired: 7 in]
            n151 = case shown="True" w780 {
              tunnel: w773 -> [w783 w795]
              tunnel: w774 -> [w784 w794]
              tunnel: [w782 w792] -> w770
              tunnel: [w781 w791] -> w769
              frame False {
                n152 = call "Read Current State Machine.vi"("error in (no error)"=w784, "Channel Manager in"=w783) -> ("error out"=w787:errorcluster, "State Machine.lvclass"=w786:refnum<class "State Machine.lvclass">, "Channel Manager out"=w790:refnum<class "Channel Manager.lvclass">)  [unwired: 7 in]
                n153 = call "Next State.vi"("error in (no error)"=w787, "New_State"=u32 0, "State Machine in"=w786) -> ("error out"=w788:errorcluster, "State Machine out"=w789:refnum<class "State Machine.lvclass">)  [unwired: 7 in]
                n154 = call "Write Current State Machine.vi"("error in (no error)"=w788, "State Machine.lvclass"=w789, "Channel Manager in"=w790) -> ("error out"=w781:errorcluster, "Channel Manager out"=w782:refnum<class "Channel Manager.lvclass">)  [unwired: 7 in]
              }
              frame True {
                n155 = call "Read Current State Machine.vi"("error in (no error)"=w794, "Channel Manager in"=w795) -> ("error out"=w797:errorcluster, "State Machine.lvclass"=w796:refnum<class "State Machine.lvclass">, "Channel Manager out"=w800:refnum<class "Channel Manager.lvclass">)  [unwired: 7 in]
                n156 = call "Next State.vi"("error in (no error)"=w797, "New_State"=u32 14, "State Machine in"=w796) -> ("error out"=w798:errorcluster, "State Machine out"=w799:refnum<class "State Machine.lvclass">)  [unwired: 7 in]
                n157 = call "Write Current State Machine.vi"("error in (no error)"=w798, "State Machine.lvclass"=w799, "Channel Manager in"=w800) -> ("error out"=w791:errorcluster, "Channel Manager out"=w792:refnum<class "Channel Manager.lvclass">)  [unwired: 7 in]
              }
            }
          }
          frame 15 {
            n158 = call "Return Current RxTx.vi"("error in (no error)"=w815, "Channel Manager in"=w816) -> ("error out"=w813:errorcluster, "RxTx"=w814:refnum<class "RxTx.lvclass">, "Channel Manager out"=w812:refnum<class "Channel Manager.lvclass">)  [unwired: 7 in]
            n159 = call-dynamic "Read Interface.lvclass.vi"("error in (no error)"=w813, "RxTx in"=w814) -> ("error out"=w823:errorcluster, "Interface.lvclass"=w824:refnum<class "Interface.lvclass">, "RxTx out"=w820:refnum<class "RxTx.lvclass">)  [unwired: 7 in]
            n160 = call "Write Command.vi"("error in (no error)"=w823, "Command"="GET STATUS", "Interface in"=w824) -> ("error out"=w822:errorcluster, "Interface out"=w821:refnum<class "Interface.lvclass">)  [unwired: 7 in]
            n161 = call-dynamic "Write Interface.lvclass.vi"("error in (no error)"=w822, "Interface.lvclass"=w821, "RxTx in"=w820) -> ("error out"=w819:errorcluster, "RxTx out"=w818:refnum<class "RxTx.lvclass">)  [unwired: 7 in]
            n162 = call "Enqeue A Message.vi"("error in (no error)"=w819, "RxTx in"=w818) -> ("error out"=w801:errorcluster, "RxTx out"=w802:refnum<class "RxTx.lvclass">)  [unwired: 8 in]
            n163 = call "Write Current RxTx.vi"("error in (no error)"=w801, "RxTx"=w802, "Channel Manager in"=w812) -> ("error out"=w811:errorcluster, "Channel Manager out"=w810:refnum<class "Channel Manager.lvclass">)  [unwired: 7 in]
            n164 = call "Read Current State Machine.vi"("error in (no error)"=w811, "Channel Manager in"=w810) -> ("error out"=w808:errorcluster, "State Machine.lvclass"=w809:refnum<class "State Machine.lvclass">, "Channel Manager out"=w805:refnum<class "Channel Manager.lvclass">)  [unwired: 7 in]
            n165 = call "Next State.vi"("error in (no error)"=w808, "New_State"=u32 16, "State Machine in"=w809) -> ("error out"=w807:errorcluster, "State Machine out"=w806:refnum<class "State Machine.lvclass">)  [unwired: 7 in]
            n166 = call "Write Current State Machine.vi"("error in (no error)"=w807, "State Machine.lvclass"=w806, "Channel Manager in"=w805) -> ("error out"=w803:errorcluster, "Channel Manager out"=w804:refnum<class "Channel Manager.lvclass">)  [unwired: 7 in]
          }
          frame 16 {
            n167 = call "Return Current RxTx.vi"("error in (no error)"=w830, "Channel Manager in"=w831) -> ("error out"=w836:errorcluster, "RxTx"=w837:refnum<class "RxTx.lvclass">, "Channel Manager out"=w829:refnum<class "Channel Manager.lvclass">)  [unwired: 7 in]
            n168 = call "Deqeue B Msg.vi"("error in (no error)"=w836, "RxTx in"=w837) -> ("error out"=w835:errorcluster, "timeout?"=w826:bool, "RxTx out"=w834:refnum<class "RxTx.lvclass">)  [unwired: 7 in]
            n169 = call "Write Current RxTx.vi"("error in (no error)"=w835, "RxTx"=w834, "Channel Manager in"=w829) -> ("error out"=w833:errorcluster, "Channel Manager out"=w832:refnum<class "Channel Manager.lvclass">)  [unwired: 7 in]
            n170 = case shown="False" w826 {
              tunnel: w833 -> [w841 w857]
              tunnel: w832 -> [w840 w856]
              tunnel: [w839 w849] -> w828
              tunnel: [w838 w848] -> w827
              frame False {
                n171 = call "Read Current State Machine.vi"("error in (no error)"=w841, "Channel Manager in"=w840) -> ("error out"=w846:errorcluster, "State Machine.lvclass"=w847:refnum<class "State Machine.lvclass">, "Channel Manager out"=w843:refnum<class "Channel Manager.lvclass">)  [unwired: 7 in]
                n172 = call "Next State.vi"("error in (no error)"=w846, "New_State"=u32 3, "State Machine in"=w847) -> ("error out"=w845:errorcluster, "State Machine out"=w844:refnum<class "State Machine.lvclass">)  [unwired: 7 in]
                n173 = call "Write Current State Machine.vi"("error in (no error)"=w845, "State Machine.lvclass"=w844, "Channel Manager in"=w843) -> ("error out"=w838:errorcluster, "Channel Manager out"=w839:refnum<class "Channel Manager.lvclass">)  [unwired: 7 in]
              }
              frame True {
                n174 = call "Read Current State Machine.vi"("error in (no error)"=w857, "Channel Manager in"=w856) -> ("error out"=w854:errorcluster, "State Machine.lvclass"=w855:refnum<class "State Machine.lvclass">, "Channel Manager out"=w851:refnum<class "Channel Manager.lvclass">)  [unwired: 7 in]
                n175 = call "Next State.vi"("error in (no error)"=w854, "New_State"=u32 16, "State Machine in"=w855) -> ("error out"=w853:errorcluster, "State Machine out"=w852:refnum<class "State Machine.lvclass">)  [unwired: 7 in]
                n176 = call "Write Current State Machine.vi"("error in (no error)"=w853, "State Machine.lvclass"=w852, "Channel Manager in"=w851) -> ("error out"=w848:errorcluster, "Channel Manager out"=w849:refnum<class "Channel Manager.lvclass">)  [unwired: 7 in]
              }
            }
          }
          frame 98 {
          }
          frame 17 {
            n177 = call "Return Current RxTx.vi"("error in (no error)"=w863, "Channel Manager in"=w862) -> ("error out"=w876:errorcluster, "RxTx"=w877:refnum<class "RxTx.lvclass">, "Channel Manager out"=w873:refnum<class "Channel Manager.lvclass">)  [unwired: 7 in]
            n178 = call-dynamic "Read Interface.lvclass.vi"("error in (no error)"=w876, "RxTx in"=w877) -> ("error out"=w884:errorcluster, "Interface.lvclass"=w885:refnum<class "Interface.lvclass">, "RxTx out"=w879:refnum<class "RxTx.lvclass">)  [unwired: 7 in]
            n179 = call "Write Command.vi"("error in (no error)"=w884, "Command"="WRITE CAMERA SETUP", "Interface in"=w885) -> ("error out"=w881:errorcluster, "Interface out"=w880:refnum<class "Interface.lvclass">)  [unwired: 7 in]
            n180 = call-dynamic "Write Interface.lvclass.vi"("error in (no error)"=w881, "Interface.lvclass"=w880, "RxTx in"=w879) -> ("error out"=w883:errorcluster, "RxTx out"=w882:refnum<class "RxTx.lvclass">)  [unwired: 7 in]
            n181 = call "Enqeue A Message.vi"("error in (no error)"=w883, "RxTx in"=w882) -> ("error out"=w875:errorcluster, "RxTx out"=w874:refnum<class "RxTx.lvclass">)  [unwired: 8 in]
            n182 = call "Write Current RxTx.vi"("error in (no error)"=w875, "RxTx"=w874, "Channel Manager in"=w873) -> ("error out"=w872:errorcluster, "Channel Manager out"=w871:refnum<class "Channel Manager.lvclass">)  [unwired: 7 in]
            n183 = call "Read Current State Machine.vi"("error in (no error)"=w872, "Channel Manager in"=w871) -> ("error out"=w869:errorcluster, "State Machine.lvclass"=w870:refnum<class "State Machine.lvclass">, "Channel Manager out"=w866:refnum<class "Channel Manager.lvclass">)  [unwired: 7 in]
            n184 = call "Next State.vi"("error in (no error)"=w869, "New_State"=u32 18, "State Machine in"=w870) -> ("error out"=w868:errorcluster, "State Machine out"=w867:refnum<class "State Machine.lvclass">)  [unwired: 7 in]
            n185 = call "Write Current State Machine.vi"("error in (no error)"=w868, "State Machine.lvclass"=w867, "Channel Manager in"=w866) -> ("error out"=w865:errorcluster, "Channel Manager out"=w864:refnum<class "Channel Manager.lvclass">)  [unwired: 7 in]
            n186 = call "Clean Acquisition Status Array.vi"("error in (no error)"=w865, "Channel Manager in"=w864) -> ("error out"=w860:errorcluster, "Channel Manager out"=w861:refnum<class "Channel Manager.lvclass">)  [unwired: 8 in]
          }
          frame 18 {
            n187 = call "Return Current RxTx.vi"("error in (no error)"=w890, "Channel Manager in"=w889) -> ("error out"=w902:errorcluster, "RxTx"=w903:refnum<class "RxTx.lvclass">, "Channel Manager out"=w899:refnum<class "Channel Manager.lvclass">)  [unwired: 7 in]
            n188 = call-dynamic "Read Interface.lvclass.vi"("error in (no error)"=w902, "RxTx in"=w903) -> ("error out"=w909:errorcluster, "Interface.lvclass"=w910:refnum<class "Interface.lvclass">, "RxTx out"=w904:refnum<class "RxTx.lvclass">)  [unwired: 7 in]
            n189 = call "Write Command.vi"("error in (no error)"=w909, "Command"="START ACQUISITION", "Interface in"=w910) -> ("error out"=w906:errorcluster, "Interface out"=w905:refnum<class "Interface.lvclass">)  [unwired: 7 in]
            n190 = call-dynamic "Write Interface.lvclass.vi"("error in (no error)"=w906, "Interface.lvclass"=w905, "RxTx in"=w904) -> ("error out"=w908:errorcluster, "RxTx out"=w907:refnum<class "RxTx.lvclass">)  [unwired: 7 in]
            n191 = call "Enqeue A Message.vi"("error in (no error)"=w908, "RxTx in"=w907) -> ("error out"=w901:errorcluster, "RxTx out"=w900:refnum<class "RxTx.lvclass">)  [unwired: 8 in]
            n192 = call "Write Current RxTx.vi"("error in (no error)"=w901, "RxTx"=w900, "Channel Manager in"=w899) -> ("error out"=w893:errorcluster, "Channel Manager out"=w892:refnum<class "Channel Manager.lvclass">)  [unwired: 7 in]
            n193 = call "Read Current State Machine.vi"("error in (no error)"=w893, "Channel Manager in"=w892) -> ("error out"=w897:errorcluster, "State Machine.lvclass"=w896:refnum<class "State Machine.lvclass">, "Channel Manager out"=w891:refnum<class "Channel Manager.lvclass">)  [unwired: 7 in]
            n194 = call "Next State.vi"("error in (no error)"=w897, "New_State"=u32 19, "State Machine in"=w896) -> ("error out"=w895:errorcluster, "State Machine out"=w894:refnum<class "State Machine.lvclass">)  [unwired: 7 in]
            n195 = call "Write Current State Machine.vi"("error in (no error)"=w895, "State Machine.lvclass"=w894, "Channel Manager in"=w891) -> ("error out"=w887:errorcluster, "Channel Manager out"=w888:refnum<class "Channel Manager.lvclass">)  [unwired: 7 in]
          }
          frame 19 {
            n196 = call "Return Current RxTx.vi"("error in (no error)"=w915, "Channel Manager in"=w914) -> ("error out"=w916:errorcluster, "RxTx"=w917:refnum<class "RxTx.lvclass">, "Channel Manager out"=w918:refnum<class "Channel Manager.lvclass">)  [unwired: 7 in]
            n197 = call "Deqeue B Msg.vi"("error in (no error)"=w916, "RxTx in"=w917) -> ("error out"=w919:errorcluster, "RxTx out"=w920:refnum<class "RxTx.lvclass">)  [unwired: 7 in, 1 out]
            n198 = call "Write Current RxTx.vi"("error in (no error)"=w919, "RxTx"=w920, "Channel Manager in"=w918) -> ("error out"=w912:errorcluster, "Channel Manager out"=w913:refnum<class "Channel Manager.lvclass">)  [unwired: 7 in]
          }
          frame 20 {
            n199 = call "Read SAVE IMAGE KINETIC _.vi"("error in (no error)"=w948, "Channel Manager in"=w947) -> ("error out"=w944:errorcluster, "SAVE IMAGE KINETIC ?"=w946:bool, "Channel Manager out"=w945:refnum<class "Channel Manager.lvclass">)  [unwired: 7 in]
            n200 = case shown="True" w946 {
              tunnel: w945 -> [w950 w957]
              tunnel: w944 -> [w949 w956]
              tunnel: [w949 w952] -> w935
              tunnel: [w950 w953] -> w936
              frame False {
              }
              frame True {
                n201 = call "Return Current RxTx.vi"("error in (no error)"=w956, "Channel Manager in"=w957) -> ("error out"=w960:errorcluster, "RxTx"=w959:refnum<class "RxTx.lvclass">, "Channel Manager out"=w970:refnum<class "Channel Manager.lvclass">)  [unwired: 7 in]
                n202 = call-dynamic "Read Interface.lvclass.vi"("error in (no error)"=w960, "RxTx in"=w959) -> ("error out"=w967:errorcluster, "Interface.lvclass"=w966:refnum<class "Interface.lvclass">, "RxTx out"=w965:refnum<class "RxTx.lvclass">)  [unwired: 7 in]
                n203 = call "Write Command.vi"("error in (no error)"=w967, "Command"="SAVE IMAGE KINETIC", "Interface in"=w966) -> ("error out"=w963:errorcluster, "Interface out"=w964:refnum<class "Interface.lvclass">)  [unwired: 7 in]
                n204 = call-dynamic "Write Interface.lvclass.vi"("error in (no error)"=w963, "Interface.lvclass"=w964, "RxTx in"=w965) -> ("error out"=w961:errorcluster, "RxTx out"=w962:refnum<class "RxTx.lvclass">)  [unwired: 7 in]
                n205 = call "Enqeue A Message.vi"("error in (no error)"=w961, "RxTx in"=w962) -> ("error out"=w968:errorcluster, "RxTx out"=w969:refnum<class "RxTx.lvclass">)  [unwired: 8 in]
                n206 = call "Write Current RxTx.vi"("error in (no error)"=w968, "RxTx"=w969, "Channel Manager in"=w970) -> ("error out"=w955:errorcluster, "Channel Manager out"=w954:refnum<class "Channel Manager.lvclass">)  [unwired: 7 in]
                n207 = call "Write SAVE IMAGE KINETIC _.vi"("error in (no error)"=w955, "SAVE IMAGE KINETIC ?"=FALSE, "Channel Manager in"=w954) -> ("error out"=w952:errorcluster, "Channel Manager out"=w953:refnum<class "Channel Manager.lvclass">)  [unwired: 7 in]
              }
            }
            n208 = call "Return Current RxTx.vi"("error in (no error)"=w935, "Channel Manager in"=w936) -> ("error out"=w933:errorcluster, "RxTx"=w934:refnum<class "RxTx.lvclass">, "Channel Manager out"=w924:refnum<class "Channel Manager.lvclass">)  [unwired: 7 in]
            n209 = call-dynamic "Read Interface.lvclass.vi"("error in (no error)"=w933, "RxTx in"=w934) -> ("error out"=w931:errorcluster, "Interface.lvclass"=w932:refnum<class "Interface.lvclass">, "RxTx out"=w927:refnum<class "RxTx.lvclass">)  [unwired: 7 in]
            n210 = call "Write Command.vi"("error in (no error)"=w931, "Command"="", "Interface in"=w932) -> ("error out"=w929:errorcluster, "Interface out"=w928:refnum<class "Interface.lvclass">)  [unwired: 7 in]
            n211 = call-dynamic "Write Interface.lvclass.vi"("error in (no error)"=w929, "Interface.lvclass"=w928, "RxTx in"=w927) -> ("error out"=w926:errorcluster, "RxTx out"=w925:refnum<class "RxTx.lvclass">)  [unwired: 7 in]
            n212 = call "Write Current RxTx.vi"("error in (no error)"=w926, "RxTx"=w925, "Channel Manager in"=w924) -> ("error out"=w922:errorcluster, "Channel Manager out"=w921:refnum<class "Channel Manager.lvclass">)  [unwired: 7 in]
            n213 = call "Read Current State Machine.vi"("error in (no error)"=w922, "Channel Manager in"=w921) -> ("error out"=w942:errorcluster, "State Machine.lvclass"=w943:refnum<class "State Machine.lvclass">, "Channel Manager out"=w939:refnum<class "Channel Manager.lvclass">)  [unwired: 7 in]
            n214 = call "Next State.vi"("error in (no error)"=w942, "New_State"=21, "State Machine in"=w943) -> ("error out"=w941:errorcluster, "State Machine out"=w940:refnum<class "State Machine.lvclass">)  [unwired: 7 in]
            n215 = call "Write Current State Machine.vi"("error in (no error)"=w941, "State Machine.lvclass"=w940, "Channel Manager in"=w939) -> ("error out"=w923:errorcluster, "Channel Manager out"=w937:refnum<class "Channel Manager.lvclass">)  [unwired: 7 in]
          }
          frame 21 {
            n216 = call "Return Current RxTx.vi"("error in (no error)"=w974, "Channel Manager in"=w973) -> ("error out"=w988:errorcluster, "RxTx"=w989:refnum<class "RxTx.lvclass">, "Channel Manager out"=w985:refnum<class "Channel Manager.lvclass">)  [unwired: 7 in]
            n217 = call-dynamic "Read Interface.lvclass.vi"("error in (no error)"=w988, "RxTx in"=w989) -> ("error out"=w994:errorcluster, "Interface.lvclass"=w995:refnum<class "Interface.lvclass">, "RxTx out"=w991:refnum<class "RxTx.lvclass">)  [unwired: 7 in]
            n218 = call "Write Command.vi"("error in (no error)"=w994, "Command"="CREATE CONCRETE PRODUCT KINETIC", "Interface in"=w995) -> ("error out"=w976:errorcluster, "Interface out"=w977:refnum<class "Interface.lvclass">)  [unwired: 7 in]
            n219 = call-dynamic "Write Interface.lvclass.vi"("error in (no error)"=w976, "Interface.lvclass"=w977, "RxTx in"=w991) -> ("error out"=w993:errorcluster, "RxTx out"=w992:refnum<class "RxTx.lvclass">)  [unwired: 7 in]
            n220 = call "Enqeue A Message.vi"("error in (no error)"=w993, "RxTx in"=w992) -> ("error out"=w987:errorcluster, "RxTx out"=w986:refnum<class "RxTx.lvclass">)  [unwired: 8 in]
            n221 = call "Write Current RxTx.vi"("error in (no error)"=w987, "RxTx"=w986, "Channel Manager in"=w985) -> ("error out"=w984:errorcluster, "Channel Manager out"=w983:refnum<class "Channel Manager.lvclass">)  [unwired: 7 in]
            n222 = call "Read Current State Machine.vi"("error in (no error)"=w984, "Channel Manager in"=w983) -> ("error out"=w982:errorcluster, "State Machine.lvclass"=w981:refnum<class "State Machine.lvclass">, "Channel Manager out"=w978:refnum<class "Channel Manager.lvclass">)  [unwired: 7 in]
            n223 = call "Next State.vi"("error in (no error)"=w982, "New_State"=u32 22, "State Machine in"=w981) -> ("error out"=w980:errorcluster, "State Machine out"=w979:refnum<class "State Machine.lvclass">)  [unwired: 7 in]
            n224 = call "Write Current State Machine.vi"("error in (no error)"=w980, "State Machine.lvclass"=w979, "Channel Manager in"=w978) -> ("error out"=w971:errorcluster, "Channel Manager out"=w972:refnum<class "Channel Manager.lvclass">)  [unwired: 7 in]
          }
          frame 22 {
            n225 = call "Return Current RxTx.vi"("error in (no error)"=w998, "Channel Manager in"=w999) -> ("error out"=w1008:errorcluster, "RxTx"=w1007:refnum<class "RxTx.lvclass">, "Channel Manager out"=w1011:refnum<class "Channel Manager.lvclass">)  [unwired: 7 in]
            n226 = call-dynamic "Read Interface.lvclass.vi"("error in (no error)"=w1008, "RxTx in"=w1007) -> ("error out"=w1003:errorcluster, "Interface.lvclass"=w1002:refnum<class "Interface.lvclass">, "RxTx out"=w1006:refnum<class "RxTx.lvclass">)  [unwired: 7 in]
            n227 = call "Write Command.vi"("error in (no error)"=w1003, "Command"="VERIFY ACQUISITION", "Interface in"=w1002) -> ("error out"=w1020:errorcluster, "Interface out"=w1019:refnum<class "Interface.lvclass">)  [unwired: 7 in]
            n228 = call-dynamic "Write Interface.lvclass.vi"("error in (no error)"=w1020, "Interface.lvclass"=w1019, "RxTx in"=w1006) -> ("error out"=w1004:errorcluster, "RxTx out"=w1005:refnum<class "RxTx.lvclass">)  [unwired: 7 in]
            n229 = call "Enqeue A Message.vi"("error in (no error)"=w1004, "RxTx in"=w1005) -> ("error out"=w1009:errorcluster, "RxTx out"=w1010:refnum<class "RxTx.lvclass">)  [unwired: 8 in]
            n230 = call "Write Current RxTx.vi"("error in (no error)"=w1009, "RxTx"=w1010, "Channel Manager in"=w1011) -> ("error out"=w1012:errorcluster, "Channel Manager out"=w1013:refnum<class "Channel Manager.lvclass">)  [unwired: 7 in]
            n231 = call "Read Current State Machine.vi"("error in (no error)"=w1012, "Channel Manager in"=w1013) -> ("error out"=w1014:errorcluster, "State Machine.lvclass"=w1015:refnum<class "State Machine.lvclass">, "Channel Manager out"=w1018:refnum<class "Channel Manager.lvclass">)  [unwired: 7 in]
            n232 = call "Next State.vi"("error in (no error)"=w1014, "New_State"=u32 23, "State Machine in"=w1015) -> ("error out"=w1016:errorcluster, "State Machine out"=w1017:refnum<class "State Machine.lvclass">)  [unwired: 7 in]
            n233 = call "Write Current State Machine.vi"("error in (no error)"=w1016, "State Machine.lvclass"=w1017, "Channel Manager in"=w1018) -> ("error out"=w996:errorcluster, "Channel Manager out"=w997:refnum<class "Channel Manager.lvclass">)  [unwired: 7 in]
          }
          frame 23 {
            n234 = call "Return Current RxTx.vi"("error in (no error)"=w1024, "Channel Manager in"=w1023) -> ("error out"=w1028:errorcluster, "RxTx"=w1029:refnum<class "RxTx.lvclass">, "Channel Manager out"=w1030:refnum<class "Channel Manager.lvclass">)  [unwired: 7 in]
            n235 = call "Deqeue B Msg.vi"("error in (no error)"=w1028, "RxTx in"=w1029) -> ("error out"=w1031:errorcluster, "timeout?"=w1025:bool, "RxTx out"=w1032:refnum<class "RxTx.lvclass">)  [unwired: 7 in]
            n236 = call "Write Current RxTx.vi"("error in (no error)"=w1031, "RxTx"=w1032, "Channel Manager in"=w1030) -> ("error out"=w1027:errorcluster, "Channel Manager out"=w1026:refnum<class "Channel Manager.lvclass">)  [unwired: 7 in]
            n237 = case shown="False" w1025 {
              tunnel: w1027 -> [w1036 w1043]
              tunnel: w1026 -> [w1035 w1044]
              tunnel: [w1034 w1044] -> w1022
              tunnel: [w1033 w1043] -> w1021
              frame False {
                n238 = call "Read Current State Machine.vi"("error in (no error)"=w1036, "Channel Manager in"=w1035) -> ("error out"=w1038:errorcluster, "State Machine.lvclass"=w1039:refnum<class "State Machine.lvclass">, "Channel Manager out"=w1042:refnum<class "Channel Manager.lvclass">)  [unwired: 7 in]
                n239 = call "Next State.vi"("error in (no error)"=w1038, "New_State"=u32 24, "State Machine in"=w1039) -> ("error out"=w1040:errorcluster, "State Machine out"=w1041:refnum<class "State Machine.lvclass">)  [unwired: 7 in]
                n240 = call "Write Current State Machine.vi"("error in (no error)"=w1040, "State Machine.lvclass"=w1041, "Channel Manager in"=w1042) -> ("error out"=w1033:errorcluster, "Channel Manager out"=w1034:refnum<class "Channel Manager.lvclass">)  [unwired: 7 in]
              }
              frame True {
              }
            }
          }
          frame 24 {
            n241 = call "Return Current RxTx.vi"("error in (no error)"=w1049, "Channel Manager in"=w1050) -> ("error out"=w1045:errorcluster, "RxTx"=w1046:refnum<class "RxTx.lvclass">, "Channel Manager out"=w1064:refnum<class "Channel Manager.lvclass">)  [unwired: 7 in]
            n242 = call-dynamic "Read Interface.lvclass.vi"("error in (no error)"=w1045, "RxTx in"=w1046) -> ("error out"=w1053:errorcluster, "Interface.lvclass"=w1054:refnum<class "Interface.lvclass">, "RxTx out"=w1065:refnum<class "RxTx.lvclass">)  [unwired: 7 in]
            n243 = call "Write Command.vi"("error in (no error)"=w1053, "Command"="READ ACQUIRED IMAGE KINETIC", "Interface in"=w1054) -> ("error out"=w1067:errorcluster, "Interface out"=w1066:refnum<class "Interface.lvclass">)  [unwired: 7 in]
            n244 = call-dynamic "Write Interface.lvclass.vi"("error in (no error)"=w1067, "Interface.lvclass"=w1066, "RxTx in"=w1065) -> ("error out"=w1069:errorcluster, "RxTx out"=w1068:refnum<class "RxTx.lvclass">)  [unwired: 7 in]
            n245 = call "Enqeue A Message.vi"("error in (no error)"=w1069, "RxTx in"=w1068) -> ("error out"=w1062:errorcluster, "RxTx out"=w1063:refnum<class "RxTx.lvclass">)  [unwired: 8 in]
            n246 = call "Write Current RxTx.vi"("error in (no error)"=w1062, "RxTx"=w1063, "Channel Manager in"=w1064) -> ("error out"=w1056:errorcluster, "Channel Manager out"=w1055:refnum<class "Channel Manager.lvclass">)  [unwired: 7 in]
            n247 = call "Read Current State Machine.vi"("error in (no error)"=w1056, "Channel Manager in"=w1055) -> ("error out"=w1060:errorcluster, "State Machine.lvclass"=w1061:refnum<class "State Machine.lvclass">, "Channel Manager out"=w1057:refnum<class "Channel Manager.lvclass">)  [unwired: 7 in]
            n248 = call "Next State.vi"("error in (no error)"=w1060, "New_State"=25, "State Machine in"=w1061) -> ("error out"=w1059:errorcluster, "State Machine out"=w1058:refnum<class "State Machine.lvclass">)  [unwired: 7 in]
            n249 = call "Write Current State Machine.vi"("error in (no error)"=w1059, "State Machine.lvclass"=w1058, "Channel Manager in"=w1057) -> ("error out"=w1048:errorcluster, "Channel Manager out"=w1047:refnum<class "Channel Manager.lvclass">)  [unwired: 7 in]
          }
          frame 25 {
            n250 = call "Return Current RxTx.vi"("error in (no error)"=w1073, "Channel Manager in"=w1072) -> ("error out"=w1077:errorcluster, "RxTx"=w1076:refnum<class "RxTx.lvclass">, "Channel Manager out"=w1078:refnum<class "Channel Manager.lvclass">)  [unwired: 7 in]
            n251 = call "Deqeue B Msg.vi"("error in (no error)"=w1077, "RxTx in"=w1076) -> ("error out"=w1074:errorcluster, "timeout?"=w1079:bool, "RxTx out"=w1075:refnum<class "RxTx.lvclass">)  [unwired: 7 in]
            n252 = case shown="False" w1079 {
              tunnel: w1074 -> [w1097 w1104]
              tunnel: w1075 -> [w1096 w1103]
              tunnel: w1078 -> [w1091 w1102]
              tunnel: [w1083 w1105] -> w1071
              tunnel: [w1082 w1101] -> w1070
              frame False {
                n253 = call-dynamic "Read Interface.lvclass.vi"("error in (no error)"=w1097, "RxTx in"=w1096) -> ("error out"=w1094:errorcluster, "Interface.lvclass"=w1095:refnum<class "Interface.lvclass">, "RxTx out"=w1093:refnum<class "RxTx.lvclass">)  [unwired: 7 in]
                n254 = call "Read Command.vi"("error in (no error)"=w1094, "Interface in"=w1095) -> ("error out"=w1092:errorcluster, "Command"=w1081:string)  [unwired: 7 in, 1 out]
                n255 = call "Write Current RxTx.vi"("error in (no error)"=w1092, "RxTx"=w1093, "Channel Manager in"=w1091) -> ("error out"=w1090:errorcluster, "Channel Manager out"=w1089:refnum<class "Channel Manager.lvclass">)  [unwired: 7 in]
                n256 = case shown="\"SAVE IMAGE\"" w1081 {
                  tunnel: [u32 25 ("New_State") u32 28 ("New_State") u32 26 ("New_State")] -> w1080
                  frame "fALSE", Default {
                  }
                  frame "SAVE IMAGE" {
                  }
                  frame "REPEAT" {
                  }
                }
                n257 = call "Read Current State Machine.vi"("error in (no error)"=w1090, "Channel Manager in"=w1089) -> ("error out"=w1087:errorcluster, "State Machine.lvclass"=w1088:refnum<class "State Machine.lvclass">, "Channel Manager out"=w1084:refnum<class "Channel Manager.lvclass">)  [unwired: 7 in]
                n258 = call "Next State.vi"("error in (no error)"=w1087, "New_State"=w1080, "State Machine in"=w1088) -> ("error out"=w1086:errorcluster, "State Machine out"=w1085:refnum<class "State Machine.lvclass">)  [unwired: 7 in]
                n259 = call "Write Current State Machine.vi"("error in (no error)"=w1086, "State Machine.lvclass"=w1085, "Channel Manager in"=w1084) -> ("error out"=w1082:errorcluster, "Channel Manager out"=w1083:refnum<class "Channel Manager.lvclass">)  [unwired: 7 in]
              }
              frame True {
                n260 = call "Write Current RxTx.vi"("error in (no error)"=w1104, "RxTx"=w1103, "Channel Manager in"=w1102) -> ("error out"=w1101:errorcluster, "Channel Manager out"=w1105:refnum<class "Channel Manager.lvclass">)  [unwired: 7 in]
              }
            }
          }
          frame 26 {
            n261 = call "Return Current RxTx.vi"("error in (no error)"=w1108, "Channel Manager in"=w1109) -> ("error out"=w1121:errorcluster, "RxTx"=w1122:refnum<class "RxTx.lvclass">, "Channel Manager out"=w1112:refnum<class "Channel Manager.lvclass">)  [unwired: 7 in]
            n262 = call-dynamic "Read Interface.lvclass.vi"("error in (no error)"=w1121, "RxTx in"=w1122) -> ("error out"=w1127:errorcluster, "Interface.lvclass"=w1128:refnum<class "Interface.lvclass">, "RxTx out"=w1123:refnum<class "RxTx.lvclass">)  [unwired: 7 in]
            n263 = call-dynamic "Read Abort.vi"("error in (no error)"=w1127, "Interface in"=w1128) -> ("error out"=w1124:errorcluster, "Abort"=w1126:bool, "Interface out"=w1125:refnum<class "Interface.lvclass">)  [unwired: 7 in]
            n264 = case shown="False" w1126 {
              tunnel: w1125 -> [_ w1141]
              tunnel: w1124 -> [w1130 w1140]
              tunnel: w1123 -> [w1131 w1137]
              tunnel: [w1131 w1134] -> w1113
              tunnel: [w1130 w1133] -> w1111
              tunnel: [22 27] -> w1110
              frame False {
              }
              frame True {
                n265 = call "Write Command.vi"("error in (no error)"=w1140, "Command"="ABORT ACQUISITION", "Interface in"=w1141) -> ("error out"=w1136:errorcluster, "Interface out"=w1135:refnum<class "Interface.lvclass">)  [unwired: 7 in]
                n266 = call-dynamic "Write Interface.lvclass.vi"("error in (no error)"=w1136, "Interface.lvclass"=w1135, "RxTx in"=w1137) -> ("error out"=w1138:errorcluster, "RxTx out"=w1139:refnum<class "RxTx.lvclass">)  [unwired: 7 in]
                n267 = call "Enqeue A Message.vi"("error in (no error)"=w1138, "RxTx in"=w1139) -> ("error out"=w1133:errorcluster, "RxTx out"=w1134:refnum<class "RxTx.lvclass">)  [unwired: 8 in]
              }
            }
            n268 = call "Write Current RxTx.vi"("error in (no error)"=w1111, "RxTx"=w1113, "Channel Manager in"=w1112) -> ("error out"=w1120:errorcluster, "Channel Manager out"=w1119:refnum<class "Channel Manager.lvclass">)  [unwired: 7 in]
            n269 = call "Read Current State Machine.vi"("error in (no error)"=w1120, "Channel Manager in"=w1119) -> ("error out"=w1117:errorcluster, "State Machine.lvclass"=w1118:refnum<class "State Machine.lvclass">, "Channel Manager out"=w1114:refnum<class "Channel Manager.lvclass">)  [unwired: 7 in]
            n270 = call "Next State.vi"("error in (no error)"=w1117, "New_State"=w1110, "State Machine in"=w1118) -> ("error out"=w1116:errorcluster, "State Machine out"=w1115:refnum<class "State Machine.lvclass">)  [unwired: 7 in]
            n271 = call "Write Current State Machine.vi"("error in (no error)"=w1116, "State Machine.lvclass"=w1115, "Channel Manager in"=w1114) -> ("error out"=w1106:errorcluster, "Channel Manager out"=w1107:refnum<class "Channel Manager.lvclass">)  [unwired: 7 in]
          }
          frame 27 {
            n272 = call "Return Current RxTx.vi"("error in (no error)"=w1145, "Channel Manager in"=w1146) -> ("error out"=w1153:errorcluster, "RxTx"=w1154:refnum<class "RxTx.lvclass">, "Channel Manager out"=w1149:refnum<class "Channel Manager.lvclass">)  [unwired: 7 in]
            n273 = call "Deqeue B Msg.vi"("error in (no error)"=w1153, "RxTx in"=w1154) -> ("error out"=w1151:errorcluster, "timeout?"=w1152:bool, "RxTx out"=w1150:refnum<class "RxTx.lvclass">)  [unwired: 7 in]
            n274 = call "Write Current RxTx.vi"("error in (no error)"=w1151, "RxTx"=w1150, "Channel Manager in"=w1149) -> ("error out"=w1147:errorcluster, "Channel Manager out"=w1148:refnum<class "Channel Manager.lvclass">)  [unwired: 7 in]
            n275 = case shown="False" w1152 {
              tunnel: w1148 -> [w1157 w1166]
              tunnel: w1147 -> [w1158 w1165]
              tunnel: [w1156 w1166] -> w1144
              tunnel: [w1155 w1165] -> w1143
              frame False {
                n276 = call "Read Current State Machine.vi"("error in (no error)"=w1158, "Channel Manager in"=w1157) -> ("error out"=w1160:errorcluster, "State Machine.lvclass"=w1161:refnum<class "State Machine.lvclass">, "Channel Manager out"=w1164:refnum<class "Channel Manager.lvclass">)  [unwired: 7 in]
                n277 = call "Next State.vi"("error in (no error)"=w1160, "New_State"=u32 0, "State Machine in"=w1161) -> ("error out"=w1162:errorcluster, "State Machine out"=w1163:refnum<class "State Machine.lvclass">)  [unwired: 7 in]
                n278 = call "Write Current State Machine.vi"("error in (no error)"=w1162, "State Machine.lvclass"=w1163, "Channel Manager in"=w1164) -> ("error out"=w1155:errorcluster, "Channel Manager out"=w1156:refnum<class "Channel Manager.lvclass">)  [unwired: 7 in]
              }
              frame True {
              }
            }
          }
          frame 28 {
            n279 = call "Return Current RxTx.vi"("error in (no error)"=w1188, "Channel Manager in"=w1187) -> ("error out"=w1173:errorcluster, "RxTx"=w1174:refnum<class "RxTx.lvclass">, "Channel Manager out"=w1170:refnum<class "Channel Manager.lvclass">)  [unwired: 7 in]
            n280 = call-dynamic "Read Interface.lvclass.vi"("error in (no error)"=w1173, "RxTx in"=w1174) -> ("error out"=w1178:errorcluster, "Interface.lvclass"=w1179:refnum<class "Interface.lvclass">, "RxTx out"=w1175:refnum<class "RxTx.lvclass">)  [unwired: 7 in]
            n281 = call "Write Command.vi"("error in (no error)"=w1178, "Command"="VERIFY ACQUISITION", "Interface in"=w1179) -> ("error out"=w1168:errorcluster, "Interface out"=w1169:refnum<class "Interface.lvclass">)  [unwired: 7 in]
            n282 = call-dynamic "Write Interface.lvclass.vi"("error in (no error)"=w1168, "Interface.lvclass"=w1169, "RxTx in"=w1175) -> ("error out"=w1177:errorcluster, "RxTx out"=w1176:refnum<class "RxTx.lvclass">)  [unwired: 7 in]
            n283 = call "Enqeue A Message.vi"("error in (no error)"=w1177, "RxTx in"=w1176) -> ("error out"=w1172:errorcluster, "RxTx out"=w1171:refnum<class "RxTx.lvclass">)  [unwired: 8 in]
            n284 = call "Write Current RxTx.vi"("error in (no error)"=w1172, "RxTx"=w1171, "Channel Manager in"=w1170) -> ("error out"=w1184:errorcluster, "Channel Manager out"=w1183:refnum<class "Channel Manager.lvclass">)  [unwired: 7 in]
            n285 = call "Write SAVE IMAGE KINETIC _.vi"("error in (no error)"=w1184, "SAVE IMAGE KINETIC ?"=TRUE, "Channel Manager in"=w1183) -> ("error out"=w1181:errorcluster, "Channel Manager out"=w1182:refnum<class "Channel Manager.lvclass">)  [unwired: 7 in]
            n286 = call "Read Current State Machine.vi"("error in (no error)"=w1181, "Channel Manager in"=w1182) -> ("error out"=w1194:errorcluster, "State Machine.lvclass"=w1193:refnum<class "State Machine.lvclass">, "Channel Manager out"=w1190:refnum<class "Channel Manager.lvclass">)  [unwired: 7 in]
            n287 = call "Next State.vi"("error in (no error)"=w1194, "New_State"=u32 29, "State Machine in"=w1193) -> ("error out"=w1192:errorcluster, "State Machine out"=w1191:refnum<class "State Machine.lvclass">)  [unwired: 7 in]
            n288 = call "Write Current State Machine.vi"("error in (no error)"=w1192, "State Machine.lvclass"=w1191, "Channel Manager in"=w1190) -> ("error out"=w1185:errorcluster, "Channel Manager out"=w1186:refnum<class "Channel Manager.lvclass">)  [unwired: 7 in]
          }
          frame 29 {
            n289 = call "Return Current RxTx.vi"("error in (no error)"=w1198, "Channel Manager in"=w1197) -> ("error out"=w1202:errorcluster, "RxTx"=w1203:refnum<class "RxTx.lvclass">, "Channel Manager out"=w1204:refnum<class "Channel Manager.lvclass">)  [unwired: 7 in]
            n290 = call "Deqeue B Msg.vi"("error in (no error)"=w1202, "RxTx in"=w1203) -> ("error out"=w1205:errorcluster, "timeout?"=w1199:bool, "RxTx out"=w1206:refnum<class "RxTx.lvclass">)  [unwired: 7 in]
            n291 = call "Write Current RxTx.vi"("error in (no error)"=w1205, "RxTx"=w1206, "Channel Manager in"=w1204) -> ("error out"=w1201:errorcluster, "Channel Manager out"=w1200:refnum<class "Channel Manager.lvclass">)  [unwired: 7 in]
            n292 = case shown="False" w1199 {
              tunnel: w1201 -> [w1210 w1217]
              tunnel: w1200 -> [w1209 w1218]
              tunnel: [w1208 w1218] -> w1196
              tunnel: [w1207 w1217] -> w1195
              frame False {
                n293 = call "Read Current State Machine.vi"("error in (no error)"=w1210, "Channel Manager in"=w1209) -> ("error out"=w1212:errorcluster, "State Machine.lvclass"=w1213:refnum<class "State Machine.lvclass">, "Channel Manager out"=w1216:refnum<class "Channel Manager.lvclass">)  [unwired: 7 in]
                n294 = call "Next State.vi"("error in (no error)"=w1212, "New_State"=u32 30, "State Machine in"=w1213) -> ("error out"=w1214:errorcluster, "State Machine out"=w1215:refnum<class "State Machine.lvclass">)  [unwired: 7 in]
                n295 = call "Write Current State Machine.vi"("error in (no error)"=w1214, "State Machine.lvclass"=w1215, "Channel Manager in"=w1216) -> ("error out"=w1207:errorcluster, "Channel Manager out"=w1208:refnum<class "Channel Manager.lvclass">)  [unwired: 7 in]
              }
              frame True {
              }
            }
          }
          frame 30 {
            n296 = call "Return Current RxTx.vi"("error in (no error)"=w1227, "Channel Manager in"=w1228) -> ("error out"=w1235:errorcluster, "RxTx"=w1236:refnum<class "RxTx.lvclass">, "Channel Manager out"=w1224:refnum<class "Channel Manager.lvclass">)  [unwired: 7 in]
            n297 = call-dynamic "Read Interface.lvclass.vi"("error in (no error)"=w1235, "RxTx in"=w1236) -> ("error out"=w1238:errorcluster, "Interface.lvclass"=w1237:refnum<class "Interface.lvclass">, "RxTx out"=w1219:refnum<class "RxTx.lvclass">)  [unwired: 7 in]
            n298 = call-dynamic "Read # Images.vi"("error in (no error)"=w1238, "Interface in"=w1237) -> ("error out"=w1223:errorcluster, "# Images"=w1229:u32, "Interface out"=w1222:refnum<class "Interface.lvclass">)  [unwired: 7 in]
            n299 = case shown="0" w1229 {
              tunnel: [u32 31 ("New_State") 32] -> w1239
              tunnel: w1224 -> [w1243 w1258]
              tunnel: w1223 -> [w1245 w1257]
              tunnel: w1222 -> [w1244 _]
              tunnel: [w1242 w1258] -> w1221
              tunnel: [w1241 w1257] -> w1220
              tunnel: w1219 -> [w1240 _]
              frame 0 {
                n300 = call "Write Command.vi"("error in (no error)"=w1245, "Command"="SAVE IMAGE KINETIC", "Interface in"=w1244) -> ("error out"=w1251:errorcluster, "Interface out"=w1250:refnum<class "Interface.lvclass">)  [unwired: 7 in]
                n301 = call-dynamic "Write Interface.lvclass.vi"("error in (no error)"=w1251, "Interface.lvclass"=w1250, "RxTx in"=w1240) -> ("error out"=w1253:errorcluster, "RxTx out"=w1252:refnum<class "RxTx.lvclass">)  [unwired: 7 in]
                n302 = call "Enqeue A Message.vi"("error in (no error)"=w1253, "RxTx in"=w1252) -> ("error out"=w1249:errorcluster, "RxTx out"=w1248:refnum<class "RxTx.lvclass">)  [unwired: 8 in]
                n303 = call "Write Current RxTx.vi"("error in (no error)"=w1249, "RxTx"=w1248, "Channel Manager in"=w1243) -> ("error out"=w1254:errorcluster, "Channel Manager out"=w1255:refnum<class "Channel Manager.lvclass">)  [unwired: 7 in]
                n304 = call "Write SAVE IMAGE KINETIC _.vi"("error in (no error)"=w1254, "SAVE IMAGE KINETIC ?"=FALSE, "Channel Manager in"=w1255) -> ("error out"=w1241:errorcluster, "Channel Manager out"=w1242:refnum<class "Channel Manager.lvclass">)  [unwired: 7 in]
              }
              frame 1, Default {
              }
            }
            n305 = call "Read Current State Machine.vi"("error in (no error)"=w1220, "Channel Manager in"=w1221) -> ("error out"=w1233:errorcluster, "State Machine.lvclass"=w1234:refnum<class "State Machine.lvclass">, "Channel Manager out"=w1230:refnum<class "Channel Manager.lvclass">)  [unwired: 7 in]
            n306 = call "Next State.vi"("error in (no error)"=w1233, "New_State"=w1239, "State Machine in"=w1234) -> ("error out"=w1232:errorcluster, "State Machine out"=w1231:refnum<class "State Machine.lvclass">)  [unwired: 7 in]
            n307 = call "Write Current State Machine.vi"("error in (no error)"=w1232, "State Machine.lvclass"=w1231, "Channel Manager in"=w1230) -> ("error out"=w1225:errorcluster, "Channel Manager out"=w1226:refnum<class "Channel Manager.lvclass">)  [unwired: 7 in]
          }
          frame 31 {
            n308 = call "Return Current RxTx.vi"("error in (no error)"=w1263, "Channel Manager in"=w1262) -> ("error out"=w1268:errorcluster, "RxTx"=w1269:refnum<class "RxTx.lvclass">, "Channel Manager out"=w1270:refnum<class "Channel Manager.lvclass">)  [unwired: 7 in]
            n309 = call "Deqeue B Msg.vi"("error in (no error)"=w1268, "RxTx in"=w1269) -> ("error out"=w1267:errorcluster, "timeout?"=w1271:bool, "RxTx out"=w1266:refnum<class "RxTx.lvclass">)  [unwired: 7 in]
            n310 = call "Write Current RxTx.vi"("error in (no error)"=w1267, "RxTx"=w1266, "Channel Manager in"=w1270) -> ("error out"=w1265:errorcluster, "Channel Manager out"=w1264:refnum<class "Channel Manager.lvclass">)  [unwired: 7 in]
            n311 = case shown="False" w1271 {
              tunnel: w1264 -> [w1274 w1282]
              tunnel: w1265 -> [w1275 w1283]
              tunnel: [w1273 w1282] -> w1261
              tunnel: [w1272 w1283] -> w1260
              frame False {
                n312 = call "Read Current State Machine.vi"("error in (no error)"=w1275, "Channel Manager in"=w1274) -> ("error out"=w1278:errorcluster, "State Machine.lvclass"=w1277:refnum<class "State Machine.lvclass">, "Channel Manager out"=w1281:refnum<class "Channel Manager.lvclass">)  [unwired: 7 in]
                n313 = call "Next State.vi"("error in (no error)"=w1278, "New_State"=u32 0, "State Machine in"=w1277) -> ("error out"=w1279:errorcluster, "State Machine out"=w1280:refnum<class "State Machine.lvclass">)  [unwired: 7 in]
                n314 = call "Write Current State Machine.vi"("error in (no error)"=w1279, "State Machine.lvclass"=w1280, "Channel Manager in"=w1281) -> ("error out"=w1272:errorcluster, "Channel Manager out"=w1273:refnum<class "Channel Manager.lvclass">)  [unwired: 7 in]
              }
              frame True {
              }
            }
          }
          frame 32 {
            n315 = call "Return Current RxTx.vi"("error in (no error)"=w1286, "Channel Manager in"=w1287) -> ("error out"=w1295:errorcluster, "RxTx"=w1296:refnum<class "RxTx.lvclass">, "Channel Manager out"=w1292:refnum<class "Channel Manager.lvclass">)  [unwired: 7 in]
            n316 = call-dynamic "Read Interface.lvclass.vi"("error in (no error)"=w1295, "RxTx in"=w1296) -> ("error out"=w1297:errorcluster, "Interface.lvclass"=w1299:refnum<class "Interface.lvclass">)  [unwired: 7 in, 1 out]
            n317 = call-dynamic "Read Pause Acq.vi"("error in (no error)"=w1297, "Interface in"=w1299) -> ("error out"=w1291:errorcluster, "Pause Acq"=w1298:bool)  [unwired: 7 in, 1 out]
            n318 = case shown="False" w1298 {
              tunnel: [u32 33 ("# Images") u32 32 ("# Images")] -> w1300
              frame False {
              }
              frame True {
              }
            }
            n319 = call "Read Current State Machine.vi"("error in (no error)"=w1291, "Channel Manager in"=w1292) -> ("error out"=w1294:errorcluster, "State Machine.lvclass"=w1293:refnum<class "State Machine.lvclass">, "Channel Manager out"=w1288:refnum<class "Channel Manager.lvclass">)  [unwired: 7 in]
            n320 = call "Next State.vi"("error in (no error)"=w1294, "New_State"=w1300, "State Machine in"=w1293) -> ("error out"=w1290:errorcluster, "State Machine out"=w1289:refnum<class "State Machine.lvclass">)  [unwired: 7 in]
            n321 = call "Write Current State Machine.vi"("error in (no error)"=w1290, "State Machine.lvclass"=w1289, "Channel Manager in"=w1288) -> ("error out"=w1284:errorcluster, "Channel Manager out"=w1285:refnum<class "Channel Manager.lvclass">)  [unwired: 7 in]
          }
          frame 33 {
            n322 = call "Return Current RxTx.vi"("error in (no error)"=w1305, "Channel Manager in"=w1306) -> ("error out"=w1317:errorcluster, "RxTx"=w1318:refnum<class "RxTx.lvclass">, "Channel Manager out"=w1314:refnum<class "Channel Manager.lvclass">)  [unwired: 7 in]
            n323 = call-dynamic "Read Interface.lvclass.vi"("error in (no error)"=w1317, "RxTx in"=w1318) -> ("error out"=w1323:errorcluster, "Interface.lvclass"=w1324:refnum<class "Interface.lvclass">, "RxTx out"=w1319:refnum<class "RxTx.lvclass">)  [unwired: 7 in]
            n324 = call-dynamic "Read Stop Acq.vi"("error in (no error)"=w1323, "Interface in"=w1324) -> ("error out"=w1320:errorcluster, "Stop Acq"=w1322:bool, "Interface out"=w1321:refnum<class "Interface.lvclass">)  [unwired: 7 in]
            n325 = case shown="False" w1322 {
              tunnel: w1321 -> [_ w1335]
              tunnel: w1320 -> [w1327 w1334]
              tunnel: [w1326 w1330] -> w1316
              tunnel: [u32 35 ("# Images") u32 34 ("# Images")] -> w1325
              tunnel: w1319 -> [w1326 w1333]
              tunnel: [w1327 w1329] -> w1315
              frame False {
              }
              frame True {
                n326 = call "Write Command.vi"("error in (no error)"=w1334, "Command"="STOP ACQUISITION", "Interface in"=w1335) -> ("error out"=w1332:errorcluster, "Interface out"=w1331:refnum<class "Interface.lvclass">)  [unwired: 7 in]
                n327 = call-dynamic "Write Interface.lvclass.vi"("error in (no error)"=w1332, "Interface.lvclass"=w1331, "RxTx in"=w1333) -> ("error out"=w1338:errorcluster, "RxTx out"=w1337:refnum<class "RxTx.lvclass">)  [unwired: 7 in]
                n328 = call "Enqeue A Message.vi"("error in (no error)"=w1338, "RxTx in"=w1337) -> ("error out"=w1329:errorcluster, "RxTx out"=w1330:refnum<class "RxTx.lvclass">)  [unwired: 8 in]
              }
            }
            n329 = call "Write Current RxTx.vi"("error in (no error)"=w1315, "RxTx"=w1316, "Channel Manager in"=w1314) -> ("error out"=w1313:errorcluster, "Channel Manager out"=w1312:refnum<class "Channel Manager.lvclass">)  [unwired: 7 in]
            n330 = call "Read Current State Machine.vi"("error in (no error)"=w1313, "Channel Manager in"=w1312) -> ("error out"=w1310:errorcluster, "State Machine.lvclass"=w1311:refnum<class "State Machine.lvclass">, "Channel Manager out"=w1307:refnum<class "Channel Manager.lvclass">)  [unwired: 7 in]
            n331 = call "Next State.vi"("error in (no error)"=w1310, "New_State"=w1325, "State Machine in"=w1311) -> ("error out"=w1309:errorcluster, "State Machine out"=w1308:refnum<class "State Machine.lvclass">)  [unwired: 7 in]
            n332 = call "Write Current State Machine.vi"("error in (no error)"=w1309, "State Machine.lvclass"=w1308, "Channel Manager in"=w1307) -> ("error out"=w1303:errorcluster, "Channel Manager out"=w1304:refnum<class "Channel Manager.lvclass">)  [unwired: 7 in]
          }
          frame 34 {
            n333 = call "Return Current RxTx.vi"("error in (no error)"=w1342, "Channel Manager in"=w1343) -> ("error out"=w1348:errorcluster, "RxTx"=w1349:refnum<class "RxTx.lvclass">, "Channel Manager out"=w1350:refnum<class "Channel Manager.lvclass">)  [unwired: 7 in]
            n334 = call "Deqeue B Msg.vi"("error in (no error)"=w1348, "RxTx in"=w1349) -> ("error out"=w1347:errorcluster, "timeout?"=w1351:bool, "RxTx out"=w1346:refnum<class "RxTx.lvclass">)  [unwired: 7 in]
            n335 = call "Write Current RxTx.vi"("error in (no error)"=w1347, "RxTx"=w1346, "Channel Manager in"=w1350) -> ("error out"=w1345:errorcluster, "Channel Manager out"=w1344:refnum<class "Channel Manager.lvclass">)  [unwired: 7 in]
            n336 = case shown="False" w1351 {
              tunnel: w1344 -> [w1354 w1362]
              tunnel: w1345 -> [w1355 w1363]
              tunnel: [w1353 w1362] -> w1341
              tunnel: [w1352 w1363] -> w1340
              frame False {
                n337 = call "Read Current State Machine.vi"("error in (no error)"=w1355, "Channel Manager in"=w1354) -> ("error out"=w1358:errorcluster, "State Machine.lvclass"=w1357:refnum<class "State Machine.lvclass">, "Channel Manager out"=w1361:refnum<class "Channel Manager.lvclass">)  [unwired: 7 in]
                n338 = call "Next State.vi"("error in (no error)"=w1358, "New_State"=u32 0, "State Machine in"=w1357) -> ("error out"=w1359:errorcluster, "State Machine out"=w1360:refnum<class "State Machine.lvclass">)  [unwired: 7 in]
                n339 = call "Write Current State Machine.vi"("error in (no error)"=w1359, "State Machine.lvclass"=w1360, "Channel Manager in"=w1361) -> ("error out"=w1352:errorcluster, "Channel Manager out"=w1353:refnum<class "Channel Manager.lvclass">)  [unwired: 7 in]
              }
              frame True {
              }
            }
          }
          frame 35 {
            n340 = call "Return Current RxTx.vi"("error in (no error)"=w1366, "Channel Manager in"=w1367) -> ("error out"=w1380:errorcluster, "RxTx"=w1381:refnum<class "RxTx.lvclass">, "Channel Manager out"=w1379:refnum<class "Channel Manager.lvclass">)  [unwired: 7 in]
            n341 = call-dynamic "Read Interface.lvclass.vi"("error in (no error)"=w1380, "RxTx in"=w1381) -> ("error out"=w1387:errorcluster, "Interface.lvclass"=w1388:refnum<class "Interface.lvclass">, "RxTx out"=w1384:refnum<class "RxTx.lvclass">)  [unwired: 7 in]
            n342 = call "Write Command.vi"("error in (no error)"=w1387, "Command"="GET STATUS", "Interface in"=w1388) -> ("error out"=w1386:errorcluster, "Interface out"=w1385:refnum<class "Interface.lvclass">)  [unwired: 7 in]
            n343 = call-dynamic "Write Interface.lvclass.vi"("error in (no error)"=w1386, "Interface.lvclass"=w1385, "RxTx in"=w1384) -> ("error out"=w1383:errorcluster, "RxTx out"=w1382:refnum<class "RxTx.lvclass">)  [unwired: 7 in]
            n344 = call "Enqeue A Message.vi"("error in (no error)"=w1383, "RxTx in"=w1382) -> ("error out"=w1370:errorcluster, "RxTx out"=w1371:refnum<class "RxTx.lvclass">)  [unwired: 8 in]
            n345 = call "Write Current RxTx.vi"("error in (no error)"=w1370, "RxTx"=w1371, "Channel Manager in"=w1379) -> ("error out"=w1378:errorcluster, "Channel Manager out"=w1377:refnum<class "Channel Manager.lvclass">)  [unwired: 7 in]
            n346 = call "Read Current State Machine.vi"("error in (no error)"=w1378, "Channel Manager in"=w1377) -> ("error out"=w1375:errorcluster, "State Machine.lvclass"=w1376:refnum<class "State Machine.lvclass">, "Channel Manager out"=w1372:refnum<class "Channel Manager.lvclass">)  [unwired: 7 in]
            n347 = call "Next State.vi"("error in (no error)"=w1375, "New_State"=u32 36, "State Machine in"=w1376) -> ("error out"=w1374:errorcluster, "State Machine out"=w1373:refnum<class "State Machine.lvclass">)  [unwired: 7 in]
            n348 = call "Write Current State Machine.vi"("error in (no error)"=w1374, "State Machine.lvclass"=w1373, "Channel Manager in"=w1372) -> ("error out"=w1364:errorcluster, "Channel Manager out"=w1365:refnum<class "Channel Manager.lvclass">)  [unwired: 7 in]
          }
          frame 36 {
            n349 = call "Return Current RxTx.vi"("error in (no error)"=w1391, "Channel Manager in"=w1392) -> ("error out"=w1399:errorcluster, "RxTx"=w1400:refnum<class "RxTx.lvclass">, "Channel Manager out"=w1394:refnum<class "Channel Manager.lvclass">)  [unwired: 7 in]
            n350 = call "Deqeue B Msg.vi"("error in (no error)"=w1399, "RxTx in"=w1400) -> ("error out"=w1398:errorcluster, "timeout?"=w1393:bool, "RxTx out"=w1397:refnum<class "RxTx.lvclass">)  [unwired: 7 in]
            n351 = call "Write Current RxTx.vi"("error in (no error)"=w1398, "RxTx"=w1397, "Channel Manager in"=w1394) -> ("error out"=w1396:errorcluster, "Channel Manager out"=w1395:refnum<class "Channel Manager.lvclass">)  [unwired: 7 in]
            n352 = case shown="False" w1393 {
              tunnel: w1396 -> [w1404 w1411]
              tunnel: w1395 -> [w1403 w1412]
              tunnel: [w1402 w1412] -> w1390
              tunnel: [w1401 w1411] -> w1389
              frame False {
                n353 = call "Read Current State Machine.vi"("error in (no error)"=w1404, "Channel Manager in"=w1403) -> ("error out"=w1409:errorcluster, "State Machine.lvclass"=w1410:refnum<class "State Machine.lvclass">, "Channel Manager out"=w1406:refnum<class "Channel Manager.lvclass">)  [unwired: 7 in]
                n354 = call "Next State.vi"("error in (no error)"=w1409, "New_State"=u32 18, "State Machine in"=w1410) -> ("error out"=w1408:errorcluster, "State Machine out"=w1407:refnum<class "State Machine.lvclass">)  [unwired: 7 in]
                n355 = call "Write Current State Machine.vi"("error in (no error)"=w1408, "State Machine.lvclass"=w1407, "Channel Manager in"=w1406) -> ("error out"=w1401:errorcluster, "Channel Manager out"=w1402:refnum<class "Channel Manager.lvclass">)  [unwired: 7 in]
              }
              frame True {
              }
            }
          }
        }
      }
      n356 = call-dynamic "Write Channel Manager.lvclass.vi"("error in (no error)"=w14, "Channel Manager.lvclass"=w13, "SPARC4_AC in"=w12) -> ("error out"=w10:errorcluster, "SPARC4_AC out"=w11:refnum<class "S4ACS_GUI.lvclass">)  [unwired: 7 in]
      n357 = call-dynamic "Read Sync Mode.vi"("error in (no error)"=w10, "SPARC4_AC in"=w11) -> ("error out"=w18:errorcluster, "Sync Mode"=w19:u16, "SPARC4_AC out"=w17:refnum<class "S4ACS_GUI.lvclass">)  [unwired: 7 in]
      n358 = case shown="0, Default" w19 {
        tunnel: [w29 w91 w246 w330] -> w16
        tunnel: [w28 w92 w247 w331] -> w15
        tunnel: w18 -> [w33 w98 w254 w331]
        tunnel: w17 -> [w32 w99 w255 w330]
        frame 0, Default {
          # "Not Synchronized"
          n359 = call-dynamic "Read Channel Manager.lvclass.vi"("error in (no error)"=w33, "SPARC4_AC in"=w32) -> ("error out"=w23:errorcluster, "Channel Manager.lvclass"=w24:refnum<class "Channel Manager.lvclass">, "SPARC4_AC out"=w27:refnum<class "S4ACS_GUI.lvclass">)  [unwired: 7 in]
          n360 = call-dynamic "Read Available Cameras.vi"("error in (no error)"=w23, "Channel Manager in"=w24) -> ("error out"=w26:errorcluster, "Available Cameras"=w22:u8, "Channel Manager out"=w25:refnum<class "Channel Manager.lvclass">)  [unwired: 7 in]
          n361 = for {
            N: w22 -> [_]
            shift-right: [w39] -> w30
            shift-left: w25 -> [w36]
            shift-right: [w40] -> w31
            shift-left: w26 -> [w35]
            i -> [w34]
            n362 = call-dynamic "Write Current Camera.vi"("error in (no error)"=w35, "Current Camera"=w34, "Channel Manager in"=w36) -> ("error out"=w38:errorcluster, "Channel Manager out"=w37:refnum<class "Channel Manager.lvclass">)  [unwired: 7 in]
            n363 = call "Return Current RxTx.vi"("error in (no error)"=w38, "Channel Manager in"=w37) -> ("error out"=w48:errorcluster, "RxTx"=w49:refnum<class "RxTx.lvclass">, "Channel Manager out"=w41:refnum<class "Channel Manager.lvclass">)  [unwired: 7 in]
            n364 = call-dynamic "Read Interface.lvclass.vi"("error in (no error)"=w48, "RxTx in"=w49) -> ("error out"=w47:errorcluster, "Interface.lvclass"=w46:refnum<class "Interface.lvclass">)  [unwired: 7 in, 1 out]
            n365 = call "Read Command.vi"("error in (no error)"=w47, "Interface in"=w46) -> ("error out"=w42:errorcluster, "Command"=w44:string)  [unwired: 7 in, 1 out]
            n366 = Equal?(x=w44, y="ACQUISITION STARTED") -> (x = y?=w43:bool)
            n367 = case shown="True" w43 {
              tunnel: w42 -> [w51 w60]
              tunnel: [w50 w62] -> w39
              tunnel: [w51 w61] -> w40
              tunnel: w41 -> [w50 w59]
              frame False {
              }
              frame True {
                n368 = call "Read Sync Box.lvclass.vi"("error in (no error)"=w60, "Channel Manager in"=w59) -> ("error out"=w57:errorcluster, "Sync Box.lvclass"=w58:refnum<class "Sync Box.lvclass">, "Channel Manager out"=w54:refnum<class "Channel Manager.lvclass">)  [unwired: 7 in]
                n369 = call "Send Pulse.vi"("error in (no error)"=w57, "Sync Box in"=w58) -> ("error out"=w56:errorcluster, "Init acquisition time"=w70:dbl, "Sync Box out"=w55:refnum<class "Sync Box.lvclass">)  [unwired: 7 in]
                n370 = call "Write Sync Box.lvclass.vi"("error in (no error)"=w56, "Sync Box.lvclass"=w55, "Channel Manager in"=w54) -> ("error out"=w52:errorcluster, "Channel Manager out"=w53:refnum<class "Channel Manager.lvclass">)  [unwired: 7 in]
                n371 = call "Return Current RxTx.vi"("error in (no error)"=w52, "Channel Manager in"=w53) -> ("error out"=w79:errorcluster, "RxTx"=w83:refnum<class "RxTx.lvclass">, "Channel Manager out"=w85:refnum<class "Channel Manager.lvclass">)  [unwired: 7 in]
                n372 = call-dynamic "Read Interface.lvclass.vi"("error in (no error)"=w79, "RxTx in"=w83) -> ("error out"=w81:errorcluster, "Interface.lvclass"=w80:refnum<class "Interface.lvclass">, "RxTx out"=w82:refnum<class "RxTx.lvclass">)  [unwired: 7 in]
                n373 = call-dynamic "Write Initial Acq Time.vi"("error in (no error)"=w81, "Initial Acq Time"=w70, "Interface in"=w80) -> ("error out"=w69:errorcluster, "Interface out"=w68:refnum<class "Interface.lvclass">)  [unwired: 7 in]
                n374 = call "Read Camera Setup.vi"("error in (no error)"=w69, "Interface in"=w68) -> ("error out"=w66:errorcluster, "Camera Setup"=w65:T1, "Interface out"=w67:refnum<class "Interface.lvclass">)  [unwired: 7 in]
                n375 = Unbundle By Name(w65) -> ("Acquisition Mode"=w64:u8)
                n376 = call-dynamic "Write Interface.lvclass.vi"("error in (no error)"=w66, "Interface.lvclass"=w67, "RxTx in"=w82) -> ("error out"=w78:errorcluster, "RxTx out"=w84:refnum<class "RxTx.lvclass">)  [unwired: 7 in]
                n377 = call "Write Current RxTx.vi"("error in (no error)"=w78, "RxTx"=w84, "Channel Manager in"=w85) -> ("error out"=w72:errorcluster, "Channel Manager out"=w71:refnum<class "Channel Manager.lvclass">)  [unwired: 7 in]
                n378 = case shown="0, Default" w64 {
                  tunnel: [5 20] -> w63
                  frame 0, Default {
                  }
                  frame 3 {
                  }
                }
                n379 = call "Read Current State Machine.vi"("error in (no error)"=w72, "Channel Manager in"=w71) -> ("error out"=w77:errorcluster, "State Machine.lvclass"=w76:refnum<class "State Machine.lvclass">, "Channel Manager out"=w73:refnum<class "Channel Manager.lvclass">)  [unwired: 7 in]
                n380 = call "Next State.vi"("error in (no error)"=w77, "New_State"=w63, "State Machine in"=w76) -> ("error out"=w75:errorcluster, "State Machine out"=w74:refnum<class "State Machine.lvclass">)  [unwired: 7 in]
                n381 = call "Write Current State Machine.vi"("error in (no error)"=w75, "State Machine.lvclass"=w74, "Channel Manager in"=w73) -> ("error out"=w61:errorcluster, "Channel Manager out"=w62:refnum<class "Channel Manager.lvclass">)  [unwired: 7 in]
              }
            }
          }
          n382 = call-dynamic "Write Channel Manager.lvclass.vi"("error in (no error)"=w31, "Channel Manager.lvclass"=w30, "SPARC4_AC in"=w27) -> ("error out"=w28:errorcluster, "SPARC4_AC out"=w29:refnum<class "S4ACS_GUI.lvclass">)  [unwired: 7 in]
        }
        frame 1 {
          # "Continuous Mode"
          n383 = call-dynamic "Read Channel Manager.lvclass.vi"("error in (no error)"=w98, "SPARC4_AC in"=w99) -> ("error out"=w93:errorcluster, "Channel Manager.lvclass"=w94:refnum<class "Channel Manager.lvclass">, "SPARC4_AC out"=w88:refnum<class "S4ACS_GUI.lvclass">)  [unwired: 7 in]
          n384 = call "Verify Acquisition Status of the channels.vi"("error in (no error)"=w93, "Channel Manager in"=w94) -> ("error out"=w97:errorcluster, "Are the CHs OK ?"=w95:bool, "Channel Manager out"=w96:refnum<class "Channel Manager.lvclass">)  [unwired: 7 in]
          n385 = case shown="False" w95 {
            tunnel: [w101 w181] -> w89
            tunnel: [w100 w187] -> w90
            tunnel: w97 -> [w107 w183]
            tunnel: w96 -> [w108 w184]
            frame False {
              # "Send pulse when all the cameras are OK"
              n386 = call-dynamic "Read Available Cameras.vi"("error in (no error)"=w107, "Channel Manager in"=w108) -> ("error out"=w111:errorcluster, "Available Cameras"=w109:u8, "Channel Manager out"=w110:refnum<class "Channel Manager.lvclass">)  [unwired: 7 in]
              n387 = for {
                N: w109 -> [_]
                shift-right: [w161] -> w105
                shift-left: w110 -> [w164]
                shift-right: [w162] -> w104
                shift-left: w111 -> [w163]
                n388 = call "Return Current RxTx.vi"("error in (no error)"=w163, "Channel Manager in"=w164) -> ("error out"=w172:errorcluster, "RxTx"=w173:refnum<class "RxTx.lvclass">, "Channel Manager out"=w167:refnum<class "Channel Manager.lvclass">)  [unwired: 7 in]
                n389 = call-dynamic "Read Interface.lvclass.vi"("error in (no error)"=w172, "RxTx in"=w173) -> ("error out"=w171:errorcluster, "Interface.lvclass"=w170:refnum<class "Interface.lvclass">)  [unwired: 7 in, 1 out]
                n390 = call "Read Command.vi"("error in (no error)"=w171, "Interface in"=w170) -> ("error out"=w166:errorcluster, "Command"=w168:string)  [unwired: 7 in, 1 out]
                n391 = Equal?(x=w168, y="ACQUISITION STARTED") -> (x = y?=w165:bool)
                n392 = case shown="True" w165 {
                  selector: w165 -> [_ w176]
                  tunnel: w167 -> [w175 w180]
                  tunnel: w166 -> [w174 w179]
                  tunnel: [w174 w178] -> w162
                  tunnel: [w175 w177] -> w161
                  frame False {
                  }
                  frame True {
                    n393 = call "Write Current Acquisition Status.vi"("error in (no error)"=w179, "Acquisition Status"=w176, "Channel Manager in"=w180) -> ("error out"=w178:errorcluster, "Channel Manager out"=w177:refnum<class "Channel Manager.lvclass">)  [unwired: 7 in]
                  }
                }
              }
              n394 = call "Verify Acquisition Status of the channels.vi"("error in (no error)"=w104, "Channel Manager in"=w105) -> ("error out"=w103:errorcluster, "Are the CHs OK ?"=w106:bool, "Channel Manager out"=w102:refnum<class "Channel Manager.lvclass">)  [unwired: 7 in]
              n395 = case shown="True" w106 {
                tunnel: w103 -> [w112 w127]
                tunnel: w102 -> [w113 w126]
                tunnel: [w113 w115] -> w101
                tunnel: [w112 w114] -> w100
                frame False {
                }
                frame True {
                  n396 = call "Read Sync Box.lvclass.vi"("error in (no error)"=w127, "Channel Manager in"=w126) -> ("error out"=w124:errorcluster, "Sync Box.lvclass"=w125:refnum<class "Sync Box.lvclass">, "Channel Manager out"=w121:refnum<class "Channel Manager.lvclass">)  [unwired: 7 in]
                  n397 = call "Send Pulse.vi"("error in (no error)"=w124, "Sync Box in"=w125) -> ("error out"=w123:errorcluster, "Init acquisition time"=w128:dbl, "Sync Box out"=w122:refnum<class "Sync Box.lvclass">)  [unwired: 7 in]
                  n398 = call "Write Sync Box.lvclass.vi"("error in (no error)"=w123, "Sync Box.lvclass"=w122, "Channel Manager in"=w121) -> ("error out"=w120:errorcluster, "Channel Manager out"=w119:refnum<class "Channel Manager.lvclass">)  [unwired: 7 in]
                  n399 = call-dynamic "Read Available Cameras.vi"("error in (no error)"=w120, "Channel Manager in"=w119) -> ("error out"=w117:errorcluster, "Available Cameras"=w118:u8, "Channel Manager out"=w116:refnum<class "Channel Manager.lvclass">)  [unwired: 7 in]
                  n400 = for {
                    N: w118 -> [_]
                    tunnel: w128 -> [w143]
                    shift-right: [w135] -> w115
                    shift-left: w116 -> [w130]
                    shift-right: [w134] -> w114
                    shift-left: w117 -> [w131]
                    i -> [w129]
                    n401 = call-dynamic "Write Current Camera.vi"("error in (no error)"=w131, "Current Camera"=w129, "Channel Manager in"=w130) -> ("error out"=w133:errorcluster, "Channel Manager out"=w132:refnum<class "Channel Manager.lvclass">)  [unwired: 7 in]
                    n402 = call "Return Current RxTx.vi"("error in (no error)"=w133, "Channel Manager in"=w132) -> ("error out"=w152:errorcluster, "RxTx"=w156:refnum<class "RxTx.lvclass">, "Channel Manager out"=w158:refnum<class "Channel Manager.lvclass">)  [unwired: 7 in]
                    n403 = call-dynamic "Read Interface.lvclass.vi"("error in (no error)"=w152, "RxTx in"=w156) -> ("error out"=w154:errorcluster, "Interface.lvclass"=w153:refnum<class "Interface.lvclass">, "RxTx out"=w155:refnum<class "RxTx.lvclass">)  [unwired: 7 in]
                    n404 = call-dynamic "Write Initial Acq Time.vi"("error in (no error)"=w154, "Initial Acq Time"=w143, "Interface in"=w153) -> ("error out"=w140:errorcluster, "Interface out"=w139:refnum<class "Interface.lvclass">)  [unwired: 7 in]
                    n405 = call "Read Camera Setup.vi"("error in (no error)"=w140, "Interface in"=w139) -> ("error out"=w138:errorcluster, "Camera Setup"=w142:T1, "Interface out"=w137:refnum<class "Interface.lvclass">)  [unwired: 7 in]
                    n406 = Unbundle By Name(w142) -> ("Acquisition Mode"=w141:u8)
                    n407 = call-dynamic "Write Interface.lvclass.vi"("error in (no error)"=w138, "Interface.lvclass"=w137, "RxTx in"=w155) -> ("error out"=w151:errorcluster, "RxTx out"=w157:refnum<class "RxTx.lvclass">)  [unwired: 7 in]
                    n408 = case shown="3" w141 {
                      tunnel: [5 20] -> w136
                      frame 0, Default {
                      }
                      frame 3 {
                      }
                    }
                    n409 = call "Write Current RxTx.vi"("error in (no error)"=w151, "RxTx"=w157, "Channel Manager in"=w158) -> ("error out"=w145:errorcluster, "Channel Manager out"=w144:refnum<class "Channel Manager.lvclass">)  [unwired: 7 in]
                    n410 = call "Read Current State Machine.vi"("error in (no error)"=w145, "Channel Manager in"=w144) -> ("error out"=w150:errorcluster, "State Machine.lvclass"=w149:refnum<class "State Machine.lvclass">, "Channel Manager out"=w146:refnum<class "Channel Manager.lvclass">)  [unwired: 7 in]
                    n411 = call "Next State.vi"("error in (no error)"=w150, "New_State"=w136, "State Machine in"=w149) -> ("error out"=w148:errorcluster, "State Machine out"=w147:refnum<class "State Machine.lvclass">)  [unwired: 7 in]
                    n412 = call "Write Current State Machine.vi"("error in (no error)"=w148, "State Machine.lvclass"=w147, "Channel Manager in"=w146) -> ("error out"=w134:errorcluster, "Channel Manager out"=w135:refnum<class "Channel Manager.lvclass">)  [unwired: 7 in]
                  }
                }
              }
            }
            frame True {
              # "Send pulse when any channel is ok"
              n413 = call-dynamic "Read Available Cameras.vi"("error in (no error)"=w183, "Channel Manager in"=w184) -> ("error out"=w186:errorcluster, "Available Cameras"=w182:u8, "Channel Manager out"=w185:refnum<class "Channel Manager.lvclass">)  [unwired: 7 in]
              n414 = for {
                N: w182 -> [_]
                shift-right: [w191] -> w181
                shift-left: w185 -> [w193]
                shift-right: [w190] -> w187
                shift-left: w186 -> [w192]
                n415 = call "Return Current RxTx.vi"("error in (no error)"=w192, "Channel Manager in"=w193) -> ("error out"=w199:errorcluster, "RxTx"=w200:refnum<class "RxTx.lvclass">, "Channel Manager out"=w188:refnum<class "Channel Manager.lvclass">)  [unwired: 7 in]
                n416 = call-dynamic "Read Interface.lvclass.vi"("error in (no error)"=w199, "RxTx in"=w200) -> ("error out"=w198:errorcluster, "Interface.lvclass"=w197:refnum<class "Interface.lvclass">)  [unwired: 7 in, 1 out]
                n417 = call "Read Command.vi"("error in (no error)"=w198, "Interface in"=w197) -> ("error out"=w189:errorcluster, "Command"=w195:string)  [unwired: 7 in, 1 out]
                n418 = Equal?(x=w195, y="ACQUISITION STARTED") -> (x = y?=w194:bool)
                n419 = case shown="True" w194 {
                  tunnel: [w202 w213] -> w191
                  tunnel: [w201 w212] -> w190
                  tunnel: w189 -> [w201 w210]
                  tunnel: w188 -> [w202 w211]
                  frame False {
                  }
                  frame True {
                    n420 = call "Read Sync Box.lvclass.vi"("error in (no error)"=w210, "Channel Manager in"=w211) -> ("error out"=w208:errorcluster, "Sync Box.lvclass"=w209:refnum<class "Sync Box.lvclass">, "Channel Manager out"=w205:refnum<class "Channel Manager.lvclass">)  [unwired: 7 in]
                    n421 = call "Send Pulse.vi"("error in (no error)"=w208, "Sync Box in"=w209) -> ("error out"=w207:errorcluster, "Init acquisition time"=w221:dbl, "Sync Box out"=w206:refnum<class "Sync Box.lvclass">)  [unwired: 7 in]
                    n422 = call "Write Sync Box.lvclass.vi"("error in (no error)"=w207, "Sync Box.lvclass"=w206, "Channel Manager in"=w205) -> ("error out"=w204:errorcluster, "Channel Manager out"=w203:refnum<class "Channel Manager.lvclass">)  [unwired: 7 in]
                    n423 = call "Return Current RxTx.vi"("error in (no error)"=w204, "Channel Manager in"=w203) -> ("error out"=w230:errorcluster, "RxTx"=w234:refnum<class "RxTx.lvclass">, "Channel Manager out"=w236:refnum<class "Channel Manager.lvclass">)  [unwired: 7 in]
                    n424 = call-dynamic "Read Interface.lvclass.vi"("error in (no error)"=w230, "RxTx in"=w234) -> ("error out"=w232:errorcluster, "Interface.lvclass"=w231:refnum<class "Interface.lvclass">, "RxTx out"=w233:refnum<class "RxTx.lvclass">)  [unwired: 7 in]
                    n425 = call-dynamic "Write Initial Acq Time.vi"("error in (no error)"=w232, "Initial Acq Time"=w221, "Interface in"=w231) -> ("error out"=w217:errorcluster, "Interface out"=w216:refnum<class "Interface.lvclass">)  [unwired: 7 in]
                    n426 = call "Read Camera Setup.vi"("error in (no error)"=w217, "Interface in"=w216) -> ("error out"=w215:errorcluster, "Camera Setup"=w219:T1, "Interface out"=w214:refnum<class "Interface.lvclass">)  [unwired: 7 in]
                    n427 = Unbundle By Name(w219) -> ("Acquisition Mode"=w220:u8)
                    n428 = call-dynamic "Write Interface.lvclass.vi"("error in (no error)"=w215, "Interface.lvclass"=w214, "RxTx in"=w233) -> ("error out"=w229:errorcluster, "RxTx out"=w235:refnum<class "RxTx.lvclass">)  [unwired: 7 in]
                    n429 = call "Write Current RxTx.vi"("error in (no error)"=w229, "RxTx"=w235, "Channel Manager in"=w236) -> ("error out"=w223:errorcluster, "Channel Manager out"=w222:refnum<class "Channel Manager.lvclass">)  [unwired: 7 in]
                    n430 = case shown="0, Default" w220 {
                      tunnel: [5 20] -> w218
                      frame 0, Default {
                      }
                      frame 3 {
                      }
                    }
                    n431 = call "Read Current State Machine.vi"("error in (no error)"=w223, "Channel Manager in"=w222) -> ("error out"=w228:errorcluster, "State Machine.lvclass"=w227:refnum<class "State Machine.lvclass">, "Channel Manager out"=w224:refnum<class "Channel Manager.lvclass">)  [unwired: 7 in]
                    n432 = call "Next State.vi"("error in (no error)"=w228, "New_State"=w218, "State Machine in"=w227) -> ("error out"=w226:errorcluster, "State Machine out"=w225:refnum<class "State Machine.lvclass">)  [unwired: 7 in]
                    n433 = call "Write Current State Machine.vi"("error in (no error)"=w226, "State Machine.lvclass"=w225, "Channel Manager in"=w224) -> ("error out"=w212:errorcluster, "Channel Manager out"=w213:refnum<class "Channel Manager.lvclass">)  [unwired: 7 in]
                  }
                }
              }
            }
          }
          n434 = call-dynamic "Write Channel Manager.lvclass.vi"("error in (no error)"=w90, "Channel Manager.lvclass"=w89, "SPARC4_AC in"=w88) -> ("error out"=w92:errorcluster, "SPARC4_AC out"=w91:refnum<class "S4ACS_GUI.lvclass">)  [unwired: 7 in]
        }
        frame 2 {
          # "Aligned by the edge"
          n435 = call-dynamic "Read Channel Manager.lvclass.vi"("error in (no error)"=w254, "SPARC4_AC in"=w255) -> ("error out"=w249:errorcluster, "Channel Manager.lvclass"=w250:refnum<class "Channel Manager.lvclass">, "SPARC4_AC out"=w240:refnum<class "S4ACS_GUI.lvclass">)  [unwired: 7 in]
          n436 = call-dynamic "Read Available Cameras.vi"("error in (no error)"=w249, "Channel Manager in"=w250) -> ("error out"=w253:errorcluster, "Available Cameras"=w251:u8, "Channel Manager out"=w252:refnum<class "Channel Manager.lvclass">)  [unwired: 7 in]
          n437 = for {
            N: w251 -> [_]
            shift-right: [w313] -> w244
            shift-left: w252 -> [w308]
            shift-right: [w312] -> w245
            shift-left: w253 -> [w309]
            i -> [w307]
            n438 = call-dynamic "Write Current Camera.vi"("error in (no error)"=w309, "Current Camera"=w307, "Channel Manager in"=w308) -> ("error out"=w310:errorcluster, "Channel Manager out"=w311:refnum<class "Channel Manager.lvclass">)  [unwired: 7 in]
            n439 = call "Return Current RxTx.vi"("error in (no error)"=w310, "Channel Manager in"=w311) -> ("error out"=w321:errorcluster, "RxTx"=w322:refnum<class "RxTx.lvclass">, "Channel Manager out"=w316:refnum<class "Channel Manager.lvclass">)  [unwired: 7 in]
            n440 = call-dynamic "Read Interface.lvclass.vi"("error in (no error)"=w321, "RxTx in"=w322) -> ("error out"=w320:errorcluster, "Interface.lvclass"=w319:refnum<class "Interface.lvclass">)  [unwired: 7 in, 1 out]
            n441 = call "Read Command.vi"("error in (no error)"=w320, "Interface in"=w319) -> ("error out"=w315:errorcluster, "Command"=w317:string)  [unwired: 7 in, 1 out]
            n442 = Equal?(x=w317, y="ACQUISITION STARTED") -> (x = y?=w314:bool)
            n443 = case shown="True" w314 {
              selector: w314 -> [_ w325]
              tunnel: w316 -> [w324 w329]
              tunnel: w315 -> [w323 w328]
              tunnel: [w323 w327] -> w312
              tunnel: [w324 w326] -> w313
              frame False {
              }
              frame True {
                n444 = call "Write Current Acquisition Status.vi"("error in (no error)"=w328, "Acquisition Status"=w325, "Channel Manager in"=w329) -> ("error out"=w327:errorcluster, "Channel Manager out"=w326:refnum<class "Channel Manager.lvclass">)  [unwired: 7 in]
              }
            }
          }
          n445 = call "Verify Acquisition Status of the channels.vi"("error in (no error)"=w245, "Channel Manager in"=w244) -> ("error out"=w243:errorcluster, "Are the CHs OK ?"=w242:bool, "Channel Manager out"=w239:refnum<class "Channel Manager.lvclass">)  [unwired: 7 in]
          n446 = case shown="True" w242 {
            tunnel: [w257 w271] -> w248
            tunnel: w243 -> [w257 w270]
            tunnel: [w256 w259] -> w241
            tunnel: w239 -> [w256 w258]
            frame False {
            }
            frame True {
              n447 = call "Read Sync Box.lvclass.vi"("error in (no error)"=w270, "Channel Manager in"=w258) -> ("error out"=w268:errorcluster, "Sync Box.lvclass"=w269:refnum<class "Sync Box.lvclass">, "Channel Manager out"=w265:refnum<class "Channel Manager.lvclass">)  [unwired: 7 in]
              n448 = call "Send Pulse.vi"("error in (no error)"=w268, "Sync Box in"=w269) -> ("error out"=w267:errorcluster, "Init acquisition time"=w272:dbl, "Sync Box out"=w266:refnum<class "Sync Box.lvclass">)  [unwired: 7 in]
              n449 = call "Write Sync Box.lvclass.vi"("error in (no error)"=w267, "Sync Box.lvclass"=w266, "Channel Manager in"=w265) -> ("error out"=w264:errorcluster, "Channel Manager out"=w263:refnum<class "Channel Manager.lvclass">)  [unwired: 7 in]
              n450 = call-dynamic "Read Available Cameras.vi"("error in (no error)"=w264, "Channel Manager in"=w263) -> ("error out"=w261:errorcluster, "Available Cameras"=w262:u8, "Channel Manager out"=w260:refnum<class "Channel Manager.lvclass">)  [unwired: 7 in]
              n451 = for {
                N: w262 -> [_]
                tunnel: w272 -> [w289]
                shift-right: [w278] -> w259
                shift-left: w260 -> [w273]
                shift-right: [w279] -> w271
                shift-left: w261 -> [w274]
                i -> [w275]
                n452 = call-dynamic "Write Current Camera.vi"("error in (no error)"=w274, "Current Camera"=w275, "Channel Manager in"=w273) -> ("error out"=w277:errorcluster, "Channel Manager out"=w276:refnum<class "Channel Manager.lvclass">)  [unwired: 7 in]
                n453 = call "Return Current RxTx.vi"("error in (no error)"=w277, "Channel Manager in"=w276) -> ("error out"=w298:errorcluster, "RxTx"=w302:refnum<class "RxTx.lvclass">, "Channel Manager out"=w304:refnum<class "Channel Manager.lvclass">)  [unwired: 7 in]
                n454 = call-dynamic "Read Interface.lvclass.vi"("error in (no error)"=w298, "RxTx in"=w302) -> ("error out"=w300:errorcluster, "Interface.lvclass"=w299:refnum<class "Interface.lvclass">, "RxTx out"=w301:refnum<class "RxTx.lvclass">)  [unwired: 7 in]
                n455 = call-dynamic "Write Initial Acq Time.vi"("error in (no error)"=w300, "Initial Acq Time"=w289, "Interface in"=w299) -> ("error out"=w285:errorcluster, "Interface out"=w284:refnum<class "Interface.lvclass">)  [unwired: 7 in]
                n456 = call "Read Camera Setup.vi"("error in (no error)"=w285, "Interface in"=w284) -> ("error out"=w282:errorcluster, "Camera Setup"=w288:T1, "Interface out"=w283:refnum<class "Interface.lvclass">)  [unwired: 7 in]
                n457 = Unbundle By Name(w288) -> ("Acquisition Mode"=w287:u8)
                n458 = call-dynamic "Write Interface.lvclass.vi"("error in (no error)"=w282, "Interface.lvclass"=w283, "RxTx in"=w301) -> ("error out"=w297:errorcluster, "RxTx out"=w303:refnum<class "RxTx.lvclass">)  [unwired: 7 in]
                n459 = case shown="3" w287 {
                  tunnel: [5 20] -> w286
                  frame 0, Default {
                  }
                  frame 3 {
                  }
                }
                n460 = call "Write Current RxTx.vi"("error in (no error)"=w297, "RxTx"=w303, "Channel Manager in"=w304) -> ("error out"=w291:errorcluster, "Channel Manager out"=w290:refnum<class "Channel Manager.lvclass">)  [unwired: 7 in]
                n461 = call "Read Current State Machine.vi"("error in (no error)"=w291, "Channel Manager in"=w290) -> ("error out"=w296:errorcluster, "State Machine.lvclass"=w295:refnum<class "State Machine.lvclass">, "Channel Manager out"=w292:refnum<class "Channel Manager.lvclass">)  [unwired: 7 in]
                n462 = call "Next State.vi"("error in (no error)"=w296, "New_State"=w286, "State Machine in"=w295) -> ("error out"=w294:errorcluster, "State Machine out"=w293:refnum<class "State Machine.lvclass">)  [unwired: 7 in]
                n463 = call "Write Current State Machine.vi"("error in (no error)"=w294, "State Machine.lvclass"=w293, "Channel Manager in"=w292) -> ("error out"=w281:errorcluster, "Channel Manager out"=w280:refnum<class "Channel Manager.lvclass">)  [unwired: 7 in]
                n464 = call "Clean Acquisition Status Array.vi"("error in (no error)"=w281, "Channel Manager in"=w280) -> ("error out"=w279:errorcluster, "Channel Manager out"=w278:refnum<class "Channel Manager.lvclass">)  [unwired: 8 in]
              }
            }
          }
          n465 = call-dynamic "Write Channel Manager.lvclass.vi"("error in (no error)"=w248, "Channel Manager.lvclass"=w241, "SPARC4_AC in"=w240) -> ("error out"=w247:errorcluster, "SPARC4_AC out"=w246:refnum<class "S4ACS_GUI.lvclass">)  [unwired: 7 in]
        }
        frame 3 {
        }
      }
    }
    frame Error {
    }
  }
  "error out" <- w1
  "SPARC4_AC out" <- w2
